vi "Photon Counter 11_21_2018.vi"(8 "error in (no error)":errorcluster) -> (0 "error out":errorcluster)   [LabVIEW 2015]
uses:
  Public/Typedefs/Gate Mode.ctl
  Public/Typedefs/Discriminator Output.ctl
  <vilib>/Instr/_visa.llb/VISA GPIB Control REN Mode.ctl
  <vilib>/DAQmx/read.llb/DAQmx Read (Analog 2D DBL NChan NSamp).vi
  <vilib>/DAQmx/read.llb/DAQmx Read (Analog 1D DBL NChan 1Samp).vi
  <vilib>/DAQmx/write.llb/DAQmx Write (Analog DBL 1Chan 1Samp).vi
  <vilib>/DAQmx/create/channels.llb/DAQmx Create Channel (AI-Voltage-Basic).vi
  <vilib>/DAQmx/create/channels.llb/DAQmx Create Channel (AO-Voltage-Basic).vi
  <vilib>/Waveform/WDTFileIO.llb/Export Waveforms To Spreadsheet File (1D).vi
  <vilib>/DAQmx/miscellaneous.llb/DAQmx Fill In Error Info.vi
  SR400.lvlib
panel:
  out "Trigger":bool
  out "PMT":dbl(graph)=0.36701612740637457
  out "Wavemeter":dbl(graph)=5.385889833071226
  in  "file path":path=path "C:/Users/physics/Desktop/tessttt.xls"
  out "Scanning":bool=TRUE
  out "Scan Finished":bool
  out "Current Period":dbl=26.0
  out "Counter A":dbl(graph)
  out "Counter B":dbl(graph)
  in  "Monitor":bool
  in  "Start Scan":bool caption="Start Monitored Scan"
  in  "Stop Scan":bool
  out "Scan Start Time":timestamp=timestamp(3418301700.0437126 s since 1904-01-01)
  out "Counter A":dbl(graph)=5052.0
  out "Counter B":dbl(graph)=5104.0
  in  "Read Buffer Data":bool
  in  "Query Status Byte":bool
  out "Scan Start Time":timestamp=timestamp(3611333596.390047 s since 1904-01-01)
  in  "GPIB Address":i32=23 min=0 max=30 step=1
  in  "Stop Unmonitored Scan":bool
  in  "Disc A Mode":T1
  in  "Disc B Mode":T1
  in  "Disc B Slope":enum16{"Rise", "Fall"}(ring)
  in  "Disc A Slope":enum16{"Rise", "Fall"}(ring)
  in  "Trigger Slope":enum16{"Rise", "Fall"}(ring)
  in  "Set Gate Widths":bool
  in  "Set Gate Mode":bool
  out "Current":dbl[unit]=0.5 caption="Current Dwell Time"
  in  "Setpoint":dbl[unit]=0.5 caption="Dwell Time Target" min=0.0 max=60.0 step=0.5 format="%#_1g"
  in  "Set Dwell Time":bool
  in  "Setpoint":i32=2000 caption="Number of Periods Target" min=0 max=2000 step=1
  out "Current":dbl=2000.0 caption="Number of Periods Current"
  in  "Set # Periods":bool
  in  "Scan End Mode":enum16{"Stop", "Start"}(ring)
  in  "Disc B Lvl":dbl=-0.012 format="%#_13g"
  in  "Disc A Lvl":dbl=-0.012 format="%#_13g"
  in  "Display Mode":enum16{"Continuous", "Hold"}(ring)
  in  "Initialize":bool
  in  "Internal / External":bool
  in  "Set Count Time":bool
  in  "Counter B Input":enum16{"10 MHz", "INPUT 1", "INPUT 2", "TRIG"}(ring)=enum."INPUT 1"
  in  "Counter A Input":enum16{"10 MHz", "INPUT 1", "INPUT 2", "TRIG"}(ring)=enum."INPUT 1"
  in  "Count Mode":T2(ring)
  in  "Trigger Level":dbl=1.25 format="%#_13g"
  in  "VISA Resource Name":refnum<visa-resource-name>="GPIB0::23::INSTR"
  in  "Photon Counter SR 400":T3={"Mode"=0, "Count Time"=0.5, "Trigger Frequency"=10000000.0, "Trigger External?"=FALSE, "Gate A Mode"=1, "Gate A Width"=0.0002, "Gate A Delay"=0.0001, "Gate B Mode"=1, "Gate B Width"=0.0001, "Gate B Delay"=0.0003} {"Mode" items=["A,B For T Preset", "A-B For T Preset", "A+B For T Preset", "A For B Preset"]; "Gate A Mode" items=["CW", "Fixed"]; "Gate B Mode" items=["CW", "Fixed"]}
  out "Update visible/hidden":bool
  out "Current":T4=enum."Fixed"
  out "Current":T4=enum."Fixed"
  in  "stop":bool
  in  "Read to\nControl":bool
  in  "Read":bool
  out "Actual":dbl=200000.00000000003
  out "Actual":dbl=100000.00000000001
  in  "Target":dbl=100000.00000000001 caption="Gate A Width Percent Target"
  in  "Target":dbl=200000.00000000003 caption="Gate A Percent Target"
  in  "Gate Width: Time / Percent":bool caption="Time/Percent"
  in  "Start / Middle":bool
  in  "Setpoint":T4=enum."Fixed" caption="Gate B Mode Target"
  in  "Setpoint":T4=enum."Fixed" caption="Gate A Mode Target"
  out "Current":dbl[unit]=10000000.0 caption="Trigger Freq"
  in  "Setpoint":dbl[unit]=10000000.0 caption="Trigger Freq. Target"
  in  "Set Time & Freq.":bool
  in  "# Triggers vs Freq/Time":bool
  out "Current":dbl=5000000.0 caption="External Trigger # Cycles Current" format="%^#_6g"
  in  "Setpoint":dbl=5000000.0 format="%^#_6g"
  in  "Set # of Triggers":bool
  in  "Setpoint":dbl[unit]=0.0001 caption="Gate B Width Target"
  in  "Setpoint":dbl[unit]=0.0002 caption="Gate A Width Target"
  out "Current":dbl[unit]=0.0002 format="%^#_6g"
  out "Current":dbl[unit]=0.0001 format="%^#_6g"
  out "Current":dbl[unit]=0.0003
  out "Current":dbl[unit]=0.0001
  in  "Setpoint":dbl[unit]=0.0003
  in  "Setpoint":dbl[unit]=0.0001 caption="Gate A Delay Target"
  in  "Set Gate Delays":bool
  in  "Start Unmonitored Scan":bool
  in  "Setpoint":dbl[unit]=0.5 caption="Count Time Target" min=0.0 step=0.5 format="%#_1f"
  out "Current":dbl[unit]=0.5 caption="Count Time Current" min=0.0 max=10000.0 step=1.0 format="%#_7g"
  # "SR400 Control Panel"
  # "Setup"
  # "Gates"
  # "Acquisition"
  # "Gate B Mode"
  # "# of Periods"
  # "Count Time"
  # "Gate A Mode"
  # "Gate A Width"
  # "Gate B Width"
  # "Dwell Time"
  # "Gate A Delay"
  # "Gate B Delay"
  # "Only Save\nAfter Scan"
  # "Discriminator/Trigger"
  # "Set values and initialize.\n\nSettings you can \"live\" update w/o initialization:\n        All Gate Params\n        Count Time (Only largest sig digit used)\n        Dwell Time (Only largest sig digit used)\n        External Trigger\n        # Periods\n\nSettings without a \"Set _____\" button need to be changed by initialization.\n\nAll variables are initialized, but \"live\" params do not show current value until you press the set button for that parameter.\n\n\"Read\" sets the \"Current\" indicators to what the hardware has set.\n\n\"Read to Control\" sets the \"Setpoint\" controls to the values from \"Read\""
  # "Warning, saving data clears chart histories"
  # "External Trigger # of Cycles/Freq"
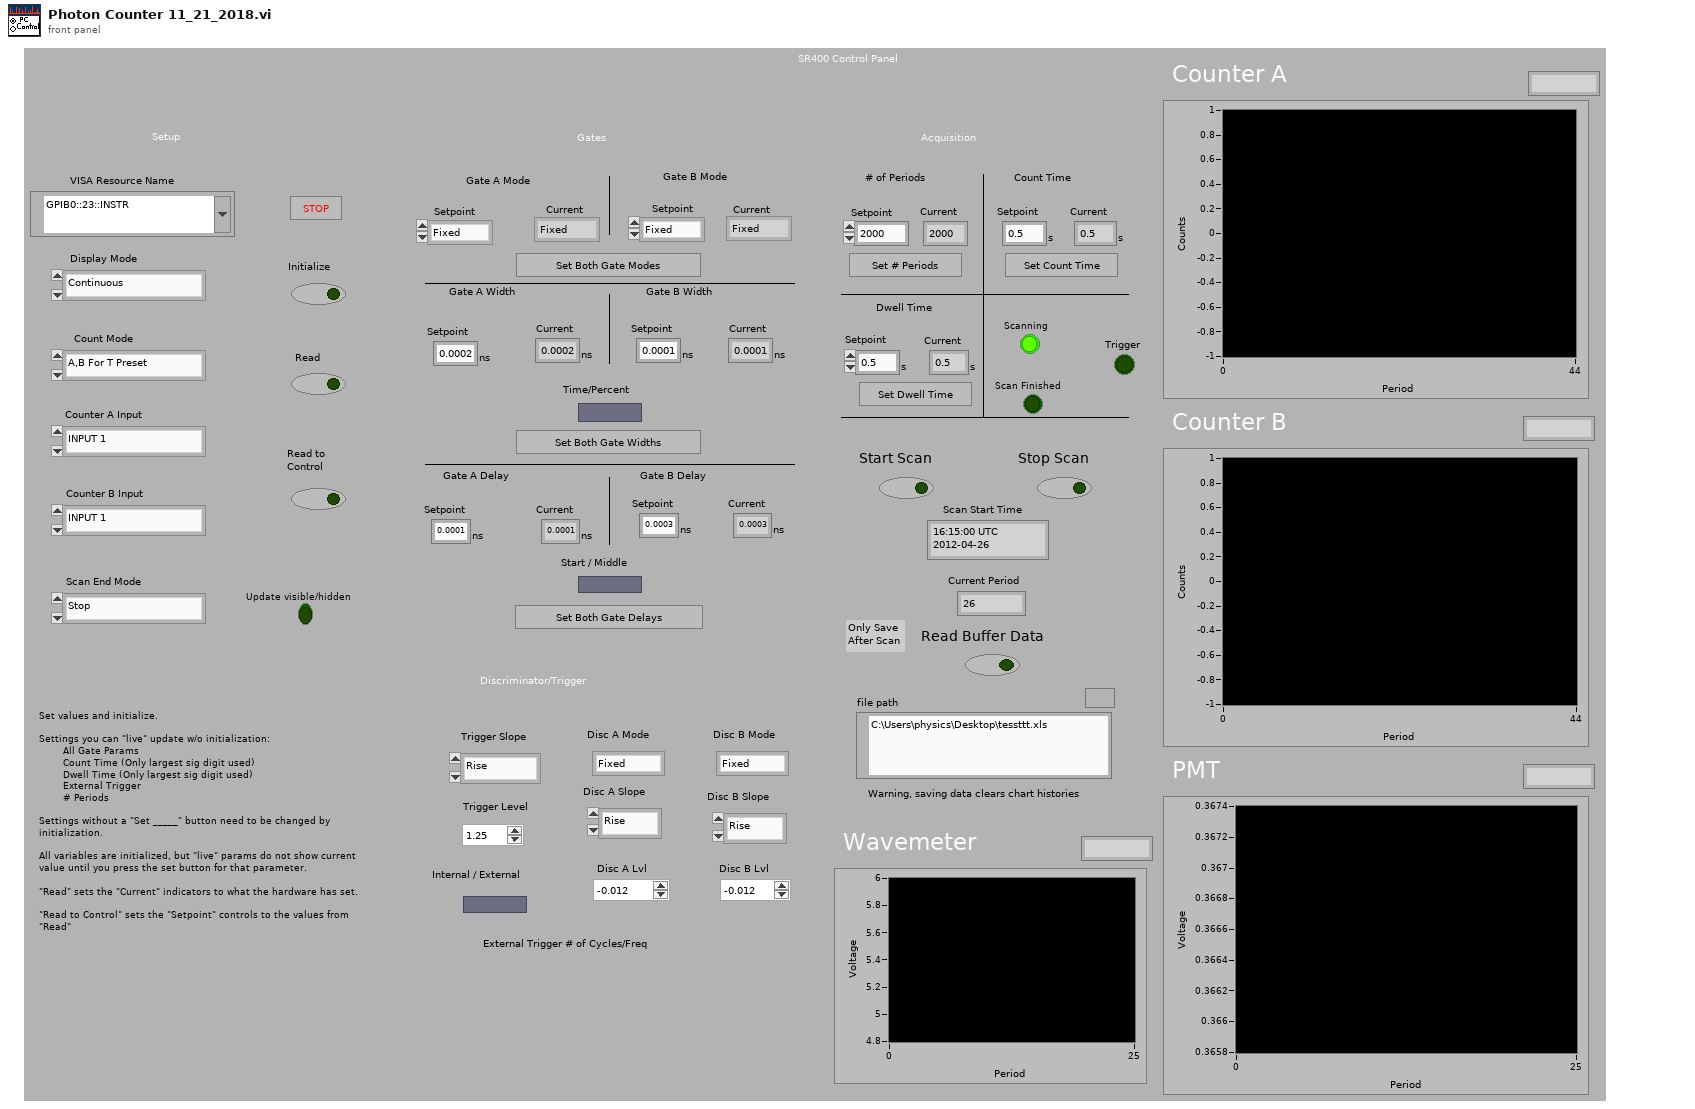
[diagram p1: front panel]
types:
  T1 = typedef "SR400.lvlib/Discriminator Output.ctl" = enum16{"Fixed", "Scan"}
  T2 = enum16{"A,B For T Preset", "A-B For T Preset", "A+B For T Preset", "A For B Preset"}
  T3 = cluster{"Mode":u16, "Count Time":dbl[unit], "Trigger Frequency":dbl[unit], "Trigger External?":bool, "Gate A Mode":u16, "Gate A Width":dbl[unit], "Gate A Delay":dbl[unit], "Gate B Mode":u16, "Gate B Width":dbl[unit], "Gate B Delay":dbl[unit]}
  T4 = typedef "SR400.lvlib/Gate Mode.ctl" = enum16{"CW", "Fixed", "Scan"}
  T5 = typedef "VISA GPIB Control REN Mode.ctl" = u16
  T6 = cluster{"Parameter Changed from front panel":bool, "Data Ready":bool, "Scan Finished":bool, "Counter Overrun":bool, "Rate Error":bool, "Recall Error":bool, "Service Request":bool, "Command Error":bool, "Triggered":bool, "Inhibited":bool, "Counting":bool}
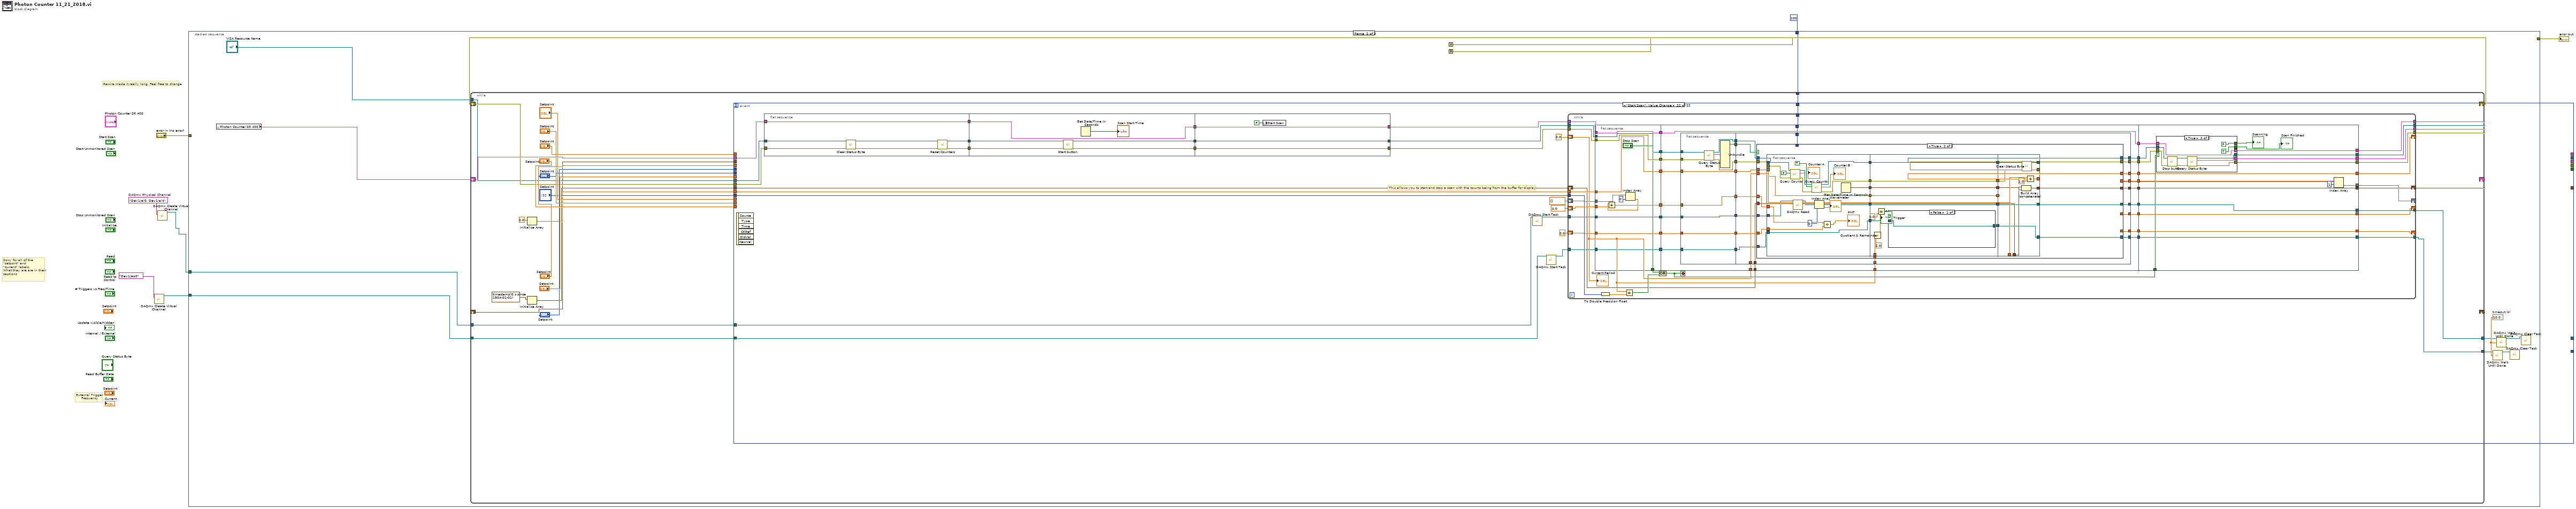
[diagram p0: block diagram]
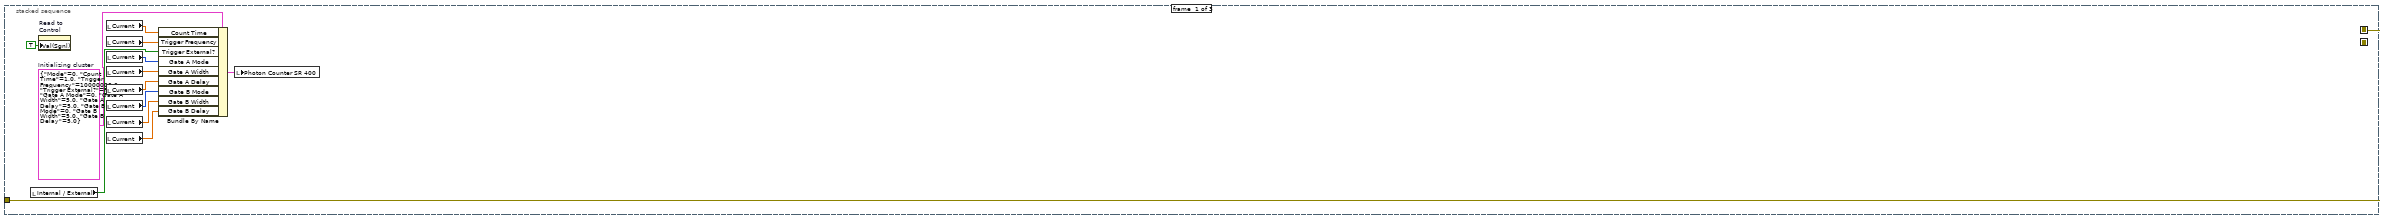
[diagram p2: hidden frame]
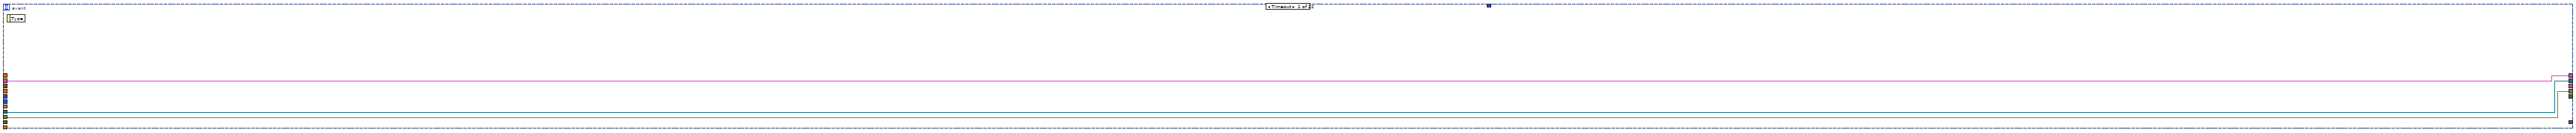
[diagram p3: hidden frame]
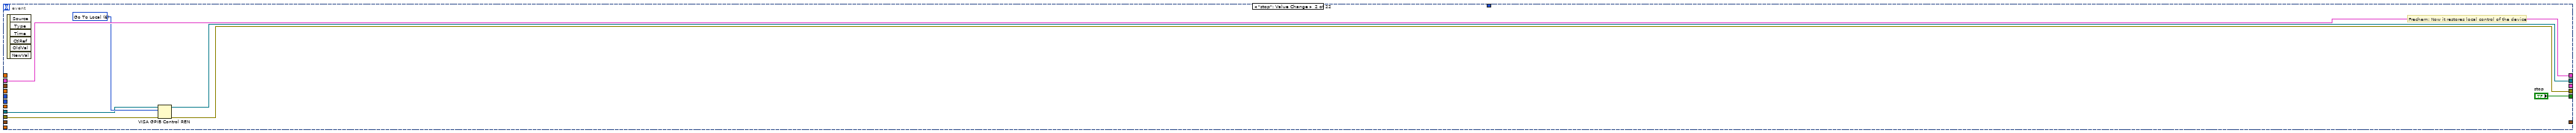
[diagram p4: hidden frame]
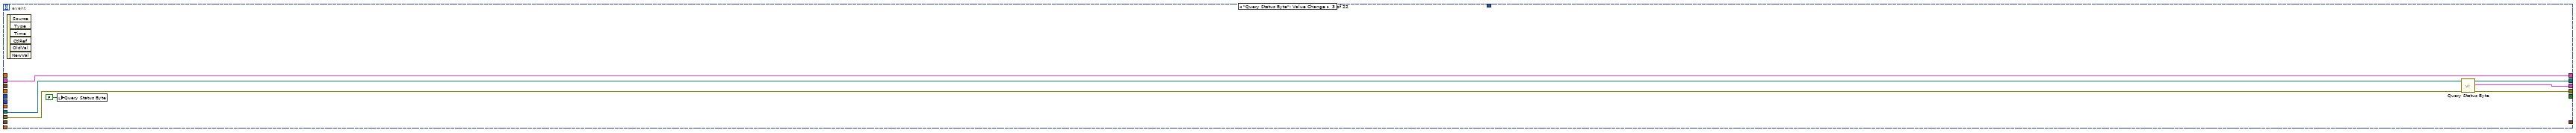
[diagram p5: hidden frame]
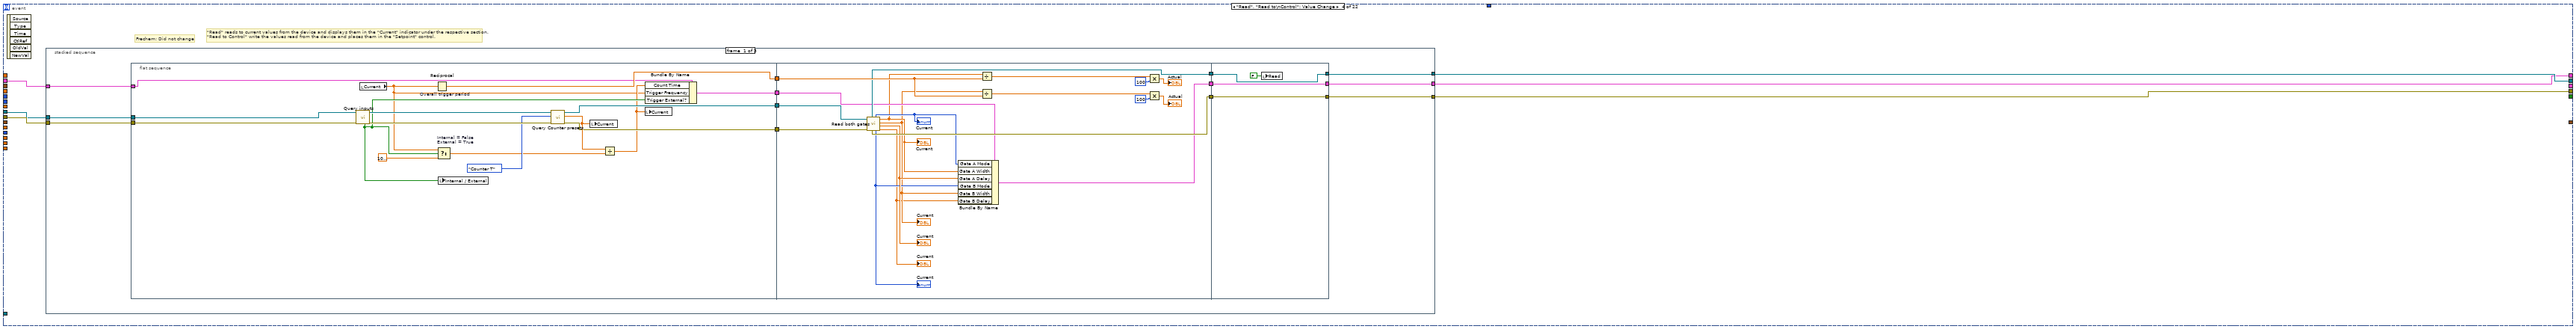
[diagram p6: hidden frame]
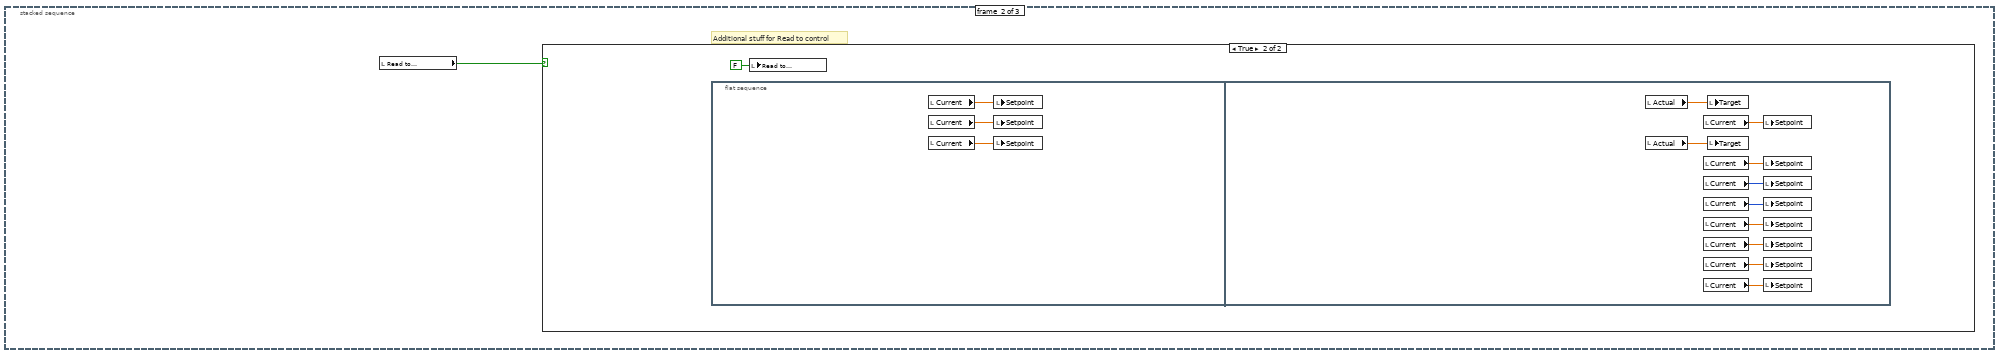
[diagram p7: hidden frame]
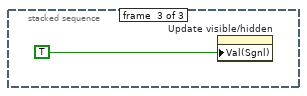
[diagram p9: hidden frame]
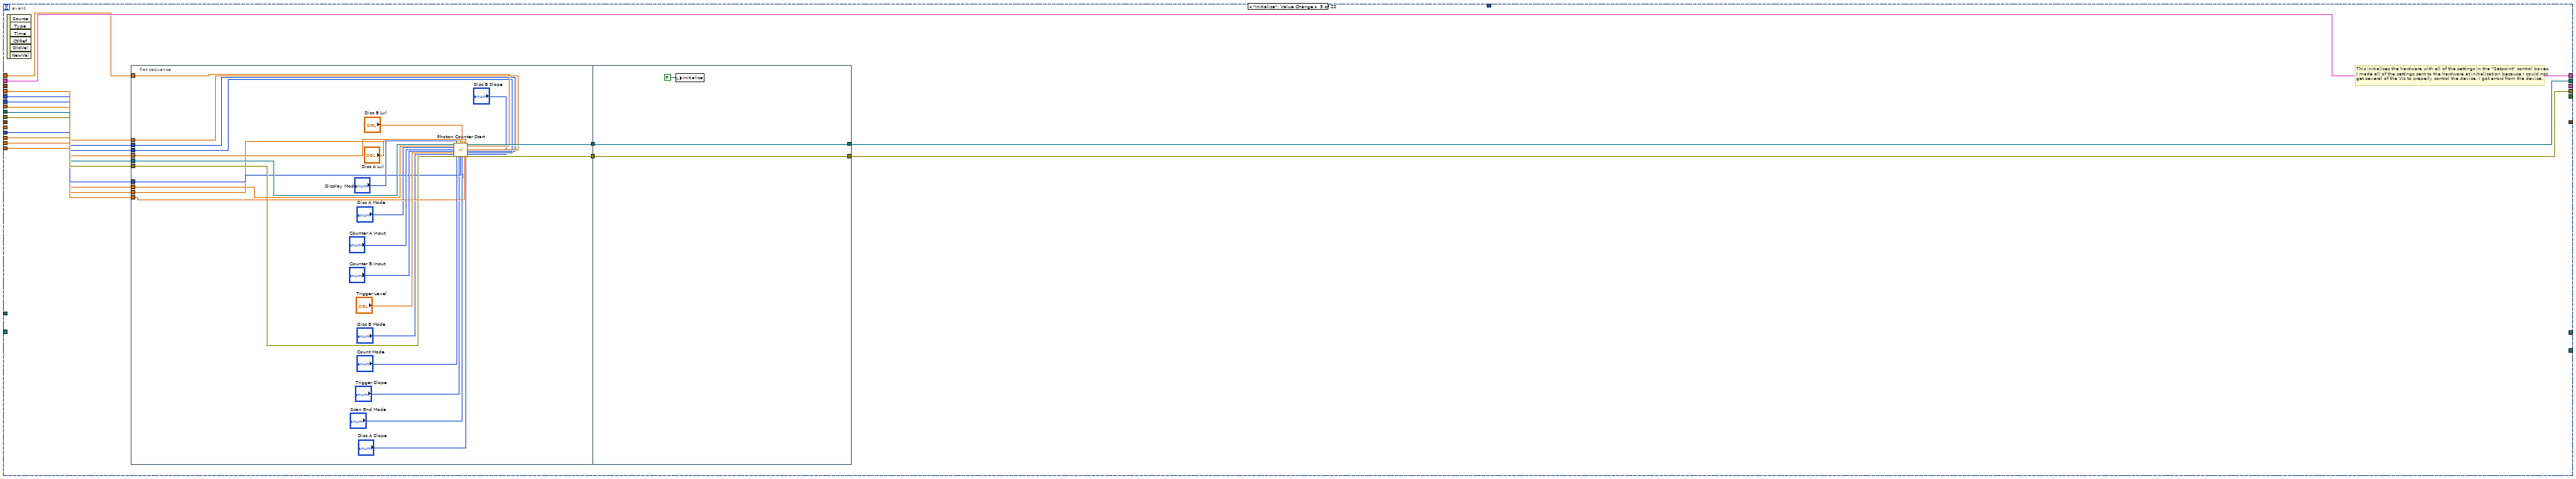
[diagram p10: hidden frame]
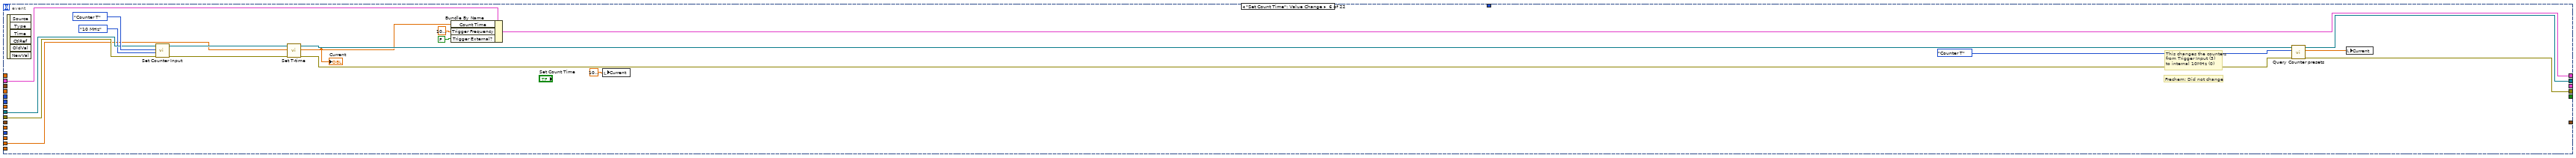
[diagram p11: hidden frame]
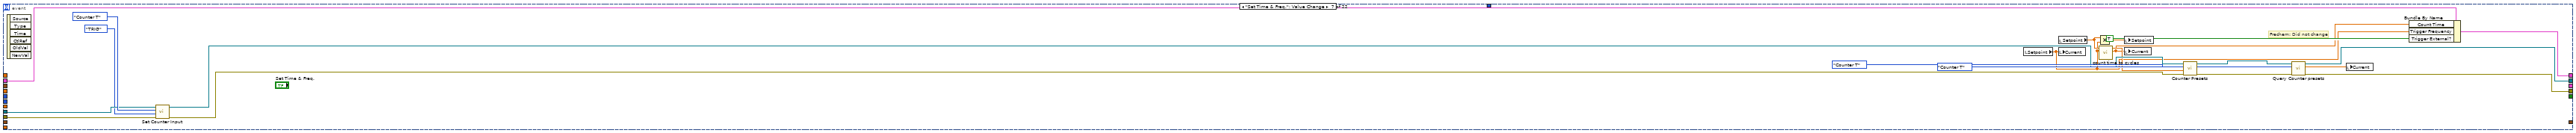
[diagram p12: hidden frame]
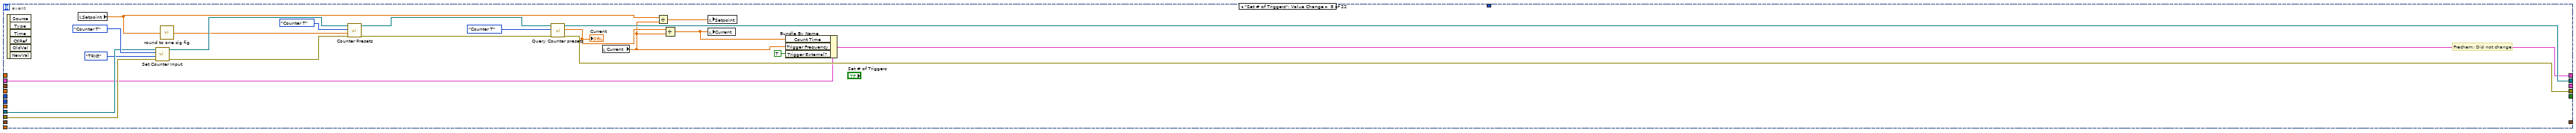
[diagram p13: hidden frame]
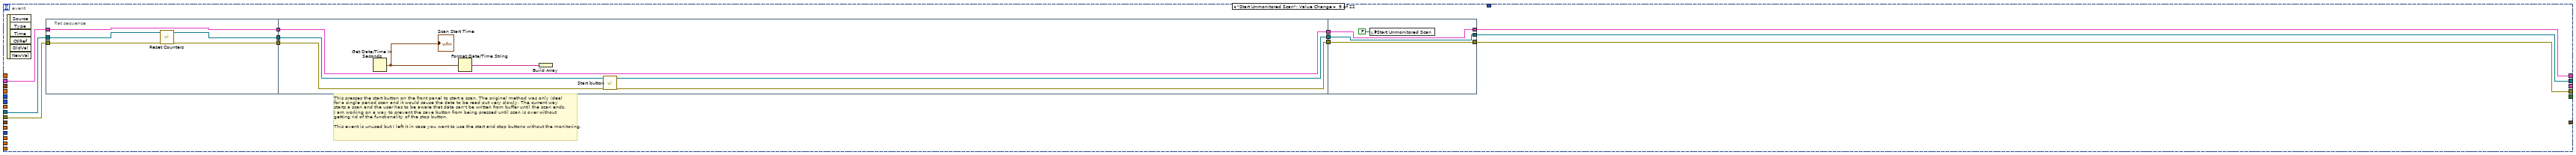
[diagram p14: hidden frame]
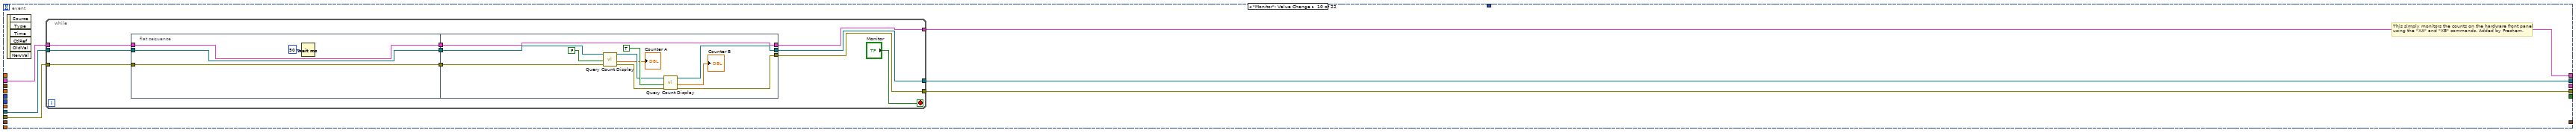
[diagram p15: hidden frame]
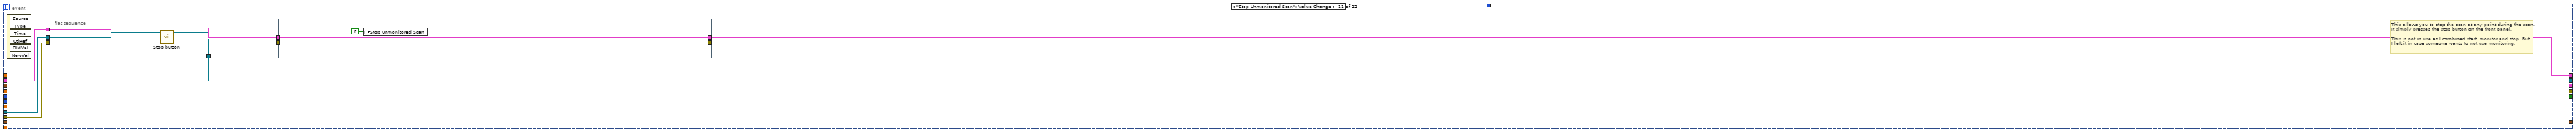
[diagram p16: hidden frame]
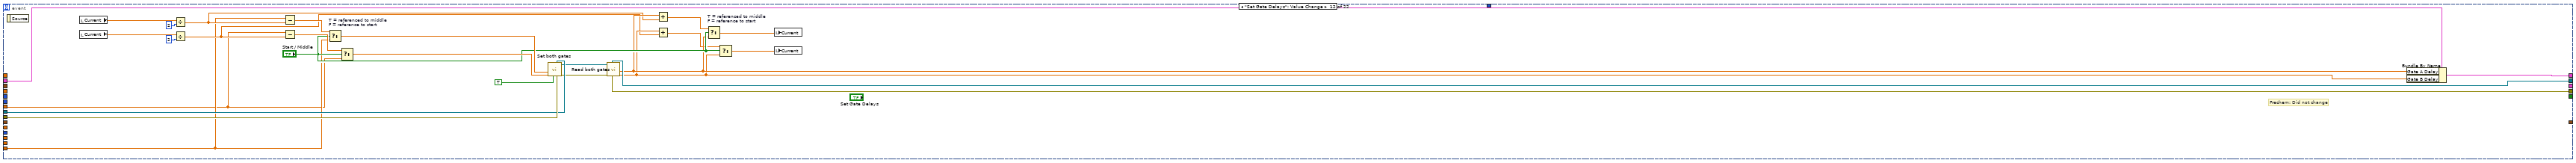
[diagram p17: hidden frame]
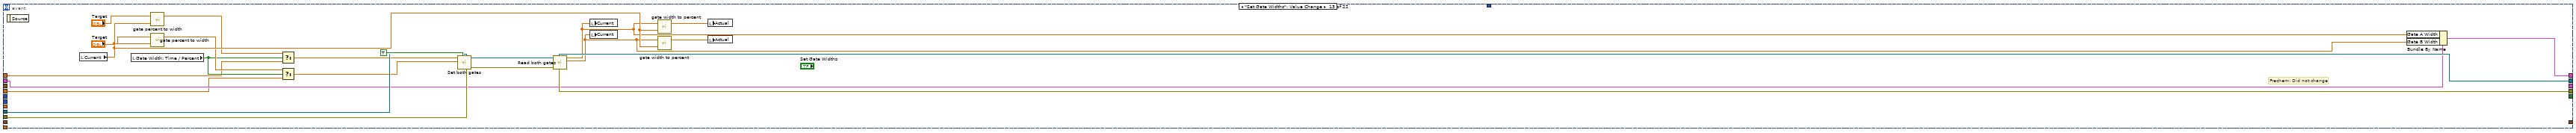
[diagram p18: hidden frame]
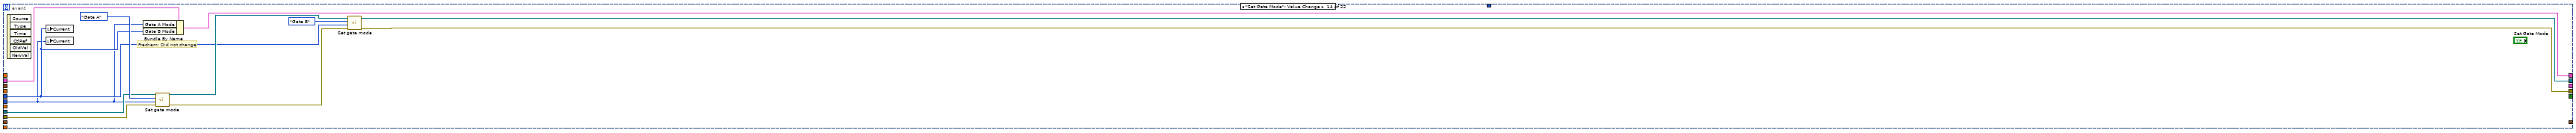
[diagram p19: hidden frame]
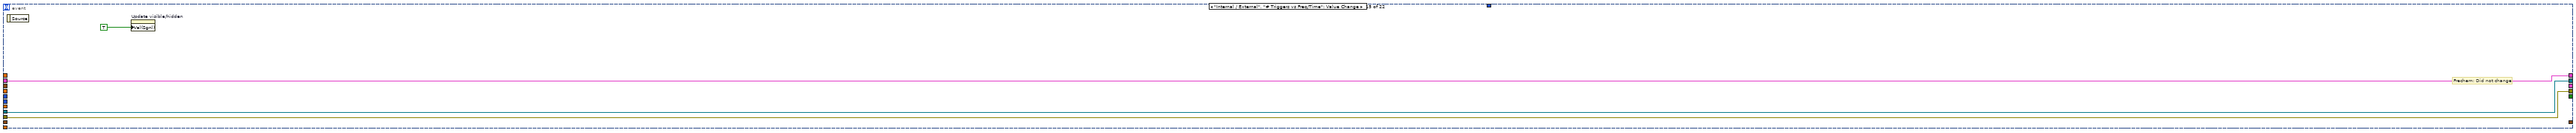
[diagram p20: hidden frame]
diagram:
  w4 = tag "Dev1/ai0, Dev1/ai4"  # DAQmx Physical Channel
  # "Rewire made it really long. Feel free to change"
  # "Sorry for all of the\n\"setpont\" and \n\"current\" labels. \nWhat they are are in their\ncaptions"
  # "External Trigger \n     Frequency"
  n1 = call-poly <vilib>:"DAQmx Create Virtual Channel.vi"("physical channels"=tag "Dev1/ao0") -> ("task out"=w1:refnum<k21>)  [unwired: 13 in, 1 out]
  n2 = call-poly <vilib>:"DAQmx Create Virtual Channel.vi"("physical channels"=w4) -> ("task out"=w3:refnum<k21>)  [unwired: 13 in, 1 out]
  n3 = stacked-sequence {
    seq-local: [w10 _ _] -> [_ w32 _]
    seq-local: [_ w31 _] -> [_ _ w874]
    tunnel: "error in (no error)" -> [w10 _ _]
    tunnel: [_ _ w874] -> w6
    tunnel: 100 ("number of samples per channel") -> [_ w28 _]
    tunnel: w3 -> [_ w27 _]
    tunnel: w1 -> [_ w26 _]
    frame #0 {
      w8 = T3 {"Mode"=0, "Count Time"=1.0, "Trigger Frequency"=10000000.0, "Trigger External?"=FALSE, "Gate A Mode"=0, "Gate A Width"=5.0, "Gate A Delay"=5.0, "Gate B Mode"=0, "Gate B Width"=5.0, "Gate B Delay"=5.0}  # Initializing cluster
      n4 = local read "Internal / External"() -> (w17:bool)
      n5 = property on="Read to\nControl" class="Bool (strict)"("Val(Sgnl)"=TRUE ("Value (Signaling)")) -> ()  [unwired: 2 in, 2 out]
      n6 = local read "Current"() -> (w19:dbl[unit])
      n7 = local read "Current"() -> (w18:dbl[unit])
      n8 = local read "Current"() -> (w16:T4)
      n9 = local read "Current"() -> (w15:dbl[unit])
      n10 = local read "Current"() -> (w14:dbl[unit])
      n11 = local read "Current"() -> (w11:T4)
      n12 = local read "Current"() -> (w12:dbl[unit])
      n13 = local read "Current"() -> (w13:dbl[unit])
      n14 = Bundle By Name(cluster=w8, "Count Time"=w19, "Trigger Frequency"=w18, "Trigger External?"=w17, "Gate A Mode"=w16, "Gate A Width"=w15, "Gate A Delay"=w14, "Gate B Mode"=w11, "Gate B Width"=w12, "Gate B Delay"=w13) -> (w9:T3)
      n15 = local write "Photon Counter SR 400"(w9) -> ()
    }
    frame #1 {
      w24 = 10.0  # timeout (s)
      n16 = local read "Photon Counter SR 400"() -> (w30:T3)
      n17 = while {
        shift-right: [w56] -> _
        shift-left: w30 -> [w55]
        shift-right: [w58] -> w31
        shift-left: w32 -> [w46]
        tunnel: "VISA Resource Name" -> [w45]
        shift-right: [w39] -> _
        shift-left: _ -> [w38]
        tunnel: w27 -> [w37]
        tunnel: w28 -> [w36]
        tunnel: w26 -> [w35]
        tunnel: [w34] -> w23
        tunnel: [w33] -> w21
        stop <- w57 stop-if-true
        n18 = Initialize Array(0.0 ("element")) -> (w42:dbl[])  [unwired: 1 in]
        n19 = Initialize Array(timestamp(0 s since 1904-01-01)) -> (w40:timestamp[])  [unwired: 1 in]
        n20 = event shown="[21] \"Start Scan\": Value Change" {
          selector: _ -> [_ _ _ _ _ _ _ _ _ _ _ _ _ _ _ _ _ _ _ _ _ _]
          dyn-events: _ -> [_ _ _ _ _ _ _ _ _ _ _ _ _ _ _ _ _ _ _ _ _ _]
          timeout: _ -> [_ _ _ _ _ _ _ _ _ _ _ _ _ _ _ _ _ _ _ _ _ _]
          tunnel: [w61 w63 w71 w80 w162 w212 w230 w254 w264 w289 w317 w344 w376 w386 w397 w400 w426 w459 w475 w482 w507 w586] -> _
          tunnel: w46 -> [w60 w66 w73 w82 w166 w203 w224 w246 w268 w288 w320 w358 w377 w390 w396 w398 w425 w458 w472 w488 w510 w589]
          tunnel: [w60 w65 w72 w79 w165 w211 w231 w253 w266 w290 _ w342 w375 w387 w396 w399 w425 w458 w474 w481 w509 w588] -> w59
          tunnel: w45 -> [w61 w64 w74 w81 w160 w204 w225 w247 w260 w287 w319 w357 w378 w391 w397 w400 w426 w459 w473 w489 w508 w590]
          tunnel: w55 -> [w62 w68 w76 w78 w161 w201 w219 w240 w262 w286 w318 w356 w364 w385 w395 w401 w427 w457 w471 w480 w506 w591]
          tunnel: [w62 w68 w76 w77 w161 w200 w218 w239 w261 w285 w316 w355 w363 w384 w395 w401 w427 w457 w471 w480 w505 w587] -> w56
          tunnel: [_ "stop" _ _ _ _ _ _ _ _ _ _ _ _ _ _ _ _ _ _ _ _] -> w57
          tunnel: "Setpoint" -> [_ _ _ _ w159 _ _ _ _ _ _ _ _ _ _ _ _ _ w470 _ w504 w582]
          tunnel: "Setpoint" -> [_ _ _ _ w158 _ _ _ _ _ _ _ w360 _ _ _ _ _ _ _ _ _]
          tunnel: "Setpoint" -> [_ _ _ _ w157 _ _ _ _ _ _ _ w359 _ _ _ _ _ _ _ _ _]
          tunnel: "Setpoint" -> [_ _ _ _ w156 _ _ _ _ _ _ w332 _ _ _ _ _ _ _ _ _ _]
          tunnel: "Setpoint" -> [_ _ _ _ w155 _ _ _ _ _ _ w331 _ _ _ _ _ _ _ _ _ _]
          tunnel: "Setpoint" -> [_ _ _ _ w154 w196 _ _ _ _ _ _ _ _ _ _ _ _ _ _ w492 _]
          tunnel: "Setpoint" -> [_ _ _ _ w152 _ _ _ _ _ _ _ _ w383 _ _ _ _ _ _ _ _]
          tunnel: "Setpoint" -> [_ _ _ _ w153 _ _ _ _ _ _ _ _ w382 _ _ _ _ _ _ _ _]
          tunnel: "Setpoint" -> [_ _ _ _ w151 _ _ _ _ _ _ _ _ _ _ _ _ _ _ w486 w493 _]
          tunnel: [_ _ w70 _ _ _ _ _ _ _ _ _ _ _ _ _ _ _ _ _ _ w585] -> _
          tunnel: w42 -> [_ _ _ _ _ _ _ _ _ _ _ _ _ _ _ _ _ _ _ _ _ w583]
          tunnel: w40 -> [_ _ _ _ _ _ _ _ _ _ _ _ _ _ _ _ _ _ _ _ _ w581]
          tunnel: [_ _ _ _ _ _ _ _ _ _ _ _ _ _ _ _ _ _ _ _ _ w580] -> w39
          tunnel: w38 -> [_ _ _ _ _ _ _ _ _ _ _ _ _ _ _ _ _ _ _ _ w494 _]
          tunnel: w37 -> [_ _ _ _ _ _ _ _ _ _ _ _ _ _ _ _ _ _ _ _ _ w575]
          tunnel: w36 -> [_ _ _ _ _ _ _ _ _ _ _ _ _ _ _ _ _ _ _ _ _ w579]
          tunnel: w35 -> [_ _ _ _ _ _ _ _ _ _ _ _ _ _ _ _ _ _ _ _ _ w573]
          tunnel: [_ _ _ _ _ _ _ _ _ _ _ _ _ _ _ _ _ _ _ _ _ w571] -> w34
          tunnel: [_ _ _ _ _ _ _ _ _ _ _ _ _ _ _ _ _ _ _ _ _ w570] -> w33
          event Timeout {
            n21 = event-data() -> ()  [unwired: 2 out]
          }
          event "stop": Value Change {
            w67 = T5 6 items=["Deassert REN", "Assert REN", "Go To Local; Deassert REN ", "Assert REN; Address Device", "Local Lockout (Addressed Devices)", "Local Lockout (This Device)", "Go To Local"] ("Mode")
            # "Frechem: Now it restores local control of the device"
            n22 = event-data() -> ()  [unwired: 7 out]
            n23 = VISA GPIB Control REN(8:w66, 10:w67, 11:w64) -> (0:w65:errorcluster, 3:w63:refnum<visa-resource-name>)
          }
          event "Query Status Byte": Value Change {
            n24 = event-data() -> ()  [unwired: 7 out]
            n25 = local write "Query Status Byte"(FALSE ("Read Channels")) -> ()
            n26 = call "Query Status Byte.vi"("error in (no error)"=w73, "VISA resource name"=w74) -> ("error out"=w72:errorcluster, "Status Register"=w70:T6, "VISA resource name out"=w71:refnum<visa-resource-name>)  [unwired: 7 in]
          }
          event "Read", "Read to\nControl": Value Change {
            # "Frechem: Did not change"
            # "\"Read\" reads to current values from the device and displays them in the \"Current\" indicator under the respective section.\n\"Read to Control\" write the values read from the device and places them in the \"Setpoint\" control."
            n27 = event-data() -> ()  [unwired: 7 out]
            n28 = stacked-sequence {
              tunnel: w82 -> [w94 _ _]
              tunnel: w81 -> [w95 _ _]
              tunnel: [w90 _ _] -> w80
              tunnel: [w88 _ _] -> w79
              tunnel: w78 -> [w86 _ _]
              tunnel: [w84 _ _] -> w77
              frame #0 {
                n29 = flat-sequence {
                  tunnel: w95 -> [w111]
                  tunnel: w94 -> [w108]
                  tunnel: [w104] -> w93
                  tunnel: [w103] -> w92
                  tunnel: [w102] -> w91
                  tunnel: w86 -> [w100]
                  tunnel: [w96] -> w85
                  tunnel: w93 -> [w124]
                  tunnel: w92 -> [w123]
                  tunnel: w91 -> [w122]
                  tunnel: [w121] -> w89
                  tunnel: [w120] -> w87
                  tunnel: w85 -> [w119]
                  tunnel: [w112] -> w83
                  tunnel: [w133] -> w90
                  tunnel: w89 -> [w133]
                  tunnel: [w132] -> w88
                  tunnel: w87 -> [w132]
                  tunnel: [w131] -> w84
                  tunnel: w83 -> [w131]
                  frame #0 {
                    n30 = call "Query inputs.vi"("error in (no error)"=w108, "VISA resource name"=w111) -> ("error out"=w109:errorcluster, "VISA resource name out"=w110:refnum<visa-resource-name>, "Externally-triggered?"=w99:bool)  [unwired: 7 out]
                    n31 = local read "Current"() -> (w97:dbl[unit])
                    n32 = Reciprocal "Overall trigger period"(x=w97) -> (1/x=w102:dbl[unit])
                    n33 = Select "Internal = False\nExternal = True"(t=w97, s=w99, f=dbl[unit] 10000000.0 ("freq")) -> (s? t:f=w106:dbl[unit])
                    n34 = local write "Internal / External"(w99) -> ()
                    n35 = call "Query Counter presets.vi"("error in (no error)"=w109, "Counter (Def: T)"=enum16{"Invalid", "Counter B", "Counter T"}."Counter T" ("i (0)"), "VISA resource name"=w110) -> ("error out"=w103:errorcluster, "Number of triggers"=w105:dbl, "VISA resource name out"=w104:refnum<visa-resource-name>)  [unwired: 6 out]
                    n36 = local write "Current"(w105) -> ()
                    n37 = Divide(x=w105, y=w106) -> (x/y=w98:dbl[unit])
                    n38 = Bundle By Name(cluster=w100, "Count Time"=w98, "Trigger Frequency"=w97, "Trigger External?"=w99) -> (w96:T3)
                    n39 = local write "Current"(w98) -> ()
                  }
                  frame #1 {
                    n40 = call "Read both gates.vi"("error in (no error)"=w123, "VISA resource name"=w124) -> ("Gate B Delay"=w113:dbl[unit], "Gate A Delay"=w116:dbl[unit], "Gate B Width"=w114:dbl[unit], "Gate A Width"=w117:dbl[unit], "Current mode B"=w115:enum16{"CW", "Fixed", "Scan"}, "Current mode A"=w118:enum16{"CW", "Fixed", "Scan"}, "error out"=w120:errorcluster, "VISA resource name out"=w121:refnum<visa-resource-name>)  [unwired: 2 out]
                    "Current" <- w114
                    "Current" <- w117
                    "Current" <- w116
                    "Current" <- w113
                    "Current" <- w118
                    "Current" <- w115
                    n41 = Bundle By Name(cluster=w119, "Gate A Mode"=w118, "Gate A Width"=w117, "Gate A Delay"=w116, "Gate B Mode"=w115, "Gate B Width"=w114, "Gate B Delay"=w113) -> (w112:T3)
                    n42 = Divide(x=w117, y=w122) -> (x/y=w126:dbl)
                    n43 = Divide(x=w114, y=w122) -> (x/y=w128:dbl)
                    n44 = Multiply(x=w126, y=i8 100) -> (x*y=→"Actual":dbl)
                    n45 = Multiply(x=w128, y=i8 100) -> (x*y=→"Actual":dbl)
                  }
                  frame #2 {
                    n46 = local write "Read"(FALSE ("Read")) -> ()
                  }
                }
              }
              frame #1 {
                # "Additional stuff for Read to control"
                n47 = local read "Read to\nControl"() -> (w135:bool)
                n48 = case shown="True" w135 {
                  frame False {
                  }
                  frame True {
                    n49 = flat-sequence {
                      frame #0 {
                        n50 = local read "Current"() -> (w138:dbl)
                        n51 = local read "Current"() -> (w137:dbl[unit])
                        n52 = local read "Current"() -> (w139:dbl[unit])
                        n53 = local write "Setpoint"(w138) -> ()
                        n54 = local write "Setpoint"(w137) -> ()
                        n55 = local write "Setpoint"(w139) -> ()
                      }
                      frame #1 {
                        n56 = local read "Actual"() -> (w146:dbl)
                        n57 = local read "Actual"() -> (w148:dbl)
                        n58 = local read "Current"() -> (w141:dbl[unit])
                        n59 = local read "Current"() -> (w142:dbl[unit])
                        n60 = local read "Current"() -> (w144:T4)
                        n61 = local read "Current"() -> (w143:T4)
                        n62 = local read "Current"() -> (w147:dbl[unit])
                        n63 = local read "Current"() -> (w145:dbl[unit])
                        n64 = local read "Current"() -> (w149:dbl[unit])
                        n65 = local read "Current"() -> (w140:dbl[unit])
                        n66 = local write "Target"(w146) -> ()
                        n67 = local write "Target"(w148) -> ()
                        n68 = local write "Setpoint"(w141) -> ()
                        n69 = local write "Setpoint"(w142) -> ()
                        n70 = local write "Setpoint"(w144) -> ()
                        n71 = local write "Setpoint"(w143) -> ()
                        n72 = local write "Setpoint"(w147) -> ()
                        n73 = local write "Setpoint"(w145) -> ()
                        n74 = local write "Setpoint"(w149) -> ()
                        n75 = local write "Setpoint"(w140) -> ()
                      }
                    }
                    n76 = local write "Read to\nControl"(FALSE ("Read to Control")) -> ()
                  }
                }
              }
              frame #2 {
                n77 = property on="Update visible/hidden" class="Bool (strict)"("Val(Sgnl)"=TRUE ("Value (Signaling)")) -> ()  [unwired: 2 in, 2 out]
              }
            }
          }
          event "Initialize": Value Change {
            # "This initializes the hardware with all of the settings in the \"Setpoint\" control boxes.\nI made all of the settings sent to the hardware at initialization because I could not \nget several of the VIs to preperly control the device. I got errors from the device."
            n78 = event-data() -> ()  [unwired: 7 out]
            n79 = flat-sequence {
              tunnel: w166 -> [w192]
              tunnel: [w191] -> w164
              tunnel: [w190] -> w163
              tunnel: w160 -> [w189]
              tunnel: w159 -> [w180]
              tunnel: w158 -> [w179]
              tunnel: w157 -> [w178]
              tunnel: w156 -> [w177]
              tunnel: w155 -> [w176]
              tunnel: w154 -> [w175]
              tunnel: w153 -> [w174]
              tunnel: w152 -> [w173]
              tunnel: w151 -> [w172]
              tunnel: [w194] -> w165
              tunnel: [w195] -> w162
              tunnel: w164 -> [w195]
              tunnel: w163 -> [w194]
              frame #0 {
                n80 = call "Photon Counter Start.vi"("VISA resource name"=w189, "Dwell Time"=w172, "Disc A Mode"="Disc A Mode", "Count A Input"="Counter A Input", "Count B Input"="Counter B Input", "Trigger Level"="Trigger Level", "Disc B Mode"="Disc B Mode", "errorIN"=w192, "Display Mode"="Display Mode", "Count Mode"="Count Mode", "Trigger Slope"="Trigger Slope", "Disc A Lvl"="Disc A Lvl", "# of periods"=w180, "Disc B Lvl"="Disc B Lvl", "Scan End Mode"="Scan End Mode", "Count Time Set"=w175, "Gate A Delay (def: 0 s)"=w177, "Gate B Delay (def: 0 s)"=w176, "Disc A\nSlope"="Disc A Slope", "Gate A Width (def: 0 s)"=w178, "Gate B Width (def: 0 s)"=w179, "Gate B Mode"=w173, "Gate A Mode"=w174, "Disc B\nSlope"="Disc B Slope") -> ("VISA resource name out"=w191:refnum<visa-resource-name>, "errorOUT"=w190:errorcluster)  [unwired: 2 in]
              }
              frame #1 {
                n81 = local write "Initialize"(FALSE ("Re-initialize")) -> ()
              }
            }
          }
          event "Set Count Time": Value Change {
            # "Frechem: Did not change"
            # "This changes the counters\nfrom Trigger Input (3)\nto internal 10MHz (0)"
            n82 = event-data() -> ()  [unwired: 7 out]
            n83 = call "Set Counter Input.vi"("error in (no error)"=w203, "Input (def: 10 MHz)"=enum16{"10 MHz", "INPUT 1", "INPUT 2", "TRIG"}."10 MHz" ("n (0.000000)"), "Counter (def: A)"=enum16{"Counter A", "Counter B", "Counter T"}."Counter T" ("i (0) 2"), "VISA resource name"=w204) -> ("error out"=w206:errorcluster, "VISA resource name out"=w205:refnum<visa-resource-name>)  [unwired: 6 out]
            n84 = call "Set T-time.vi"("errorIN"=w206, "Count Time Set"=w196, "VISA resource name"=w205) -> ("errorOUT"=w207:errorcluster, "ttimeOUT"=w199:dbl[unit], "VISA resource name out"=w210:refnum<visa-resource-name>)  [unwired: 4 out]
            "Current" <- w199
            n85 = Bundle By Name(cluster=w201, "Count Time"=w199, "Trigger Frequency"=dbl[unit] 10000000.0, "Trigger External?"=FALSE) -> (w200:T3)
            n86 = local write "Current"(dbl[unit] 10000000.0 ("freq")) -> ()
            n87 = call "Query Counter presets.vi"("error in (no error)"=w207, "Counter (Def: T)"=enum16{"Invalid", "Counter B", "Counter T"}."Counter T" ("i (0)"), "VISA resource name"=w210) -> ("error out"=w211:errorcluster, "Number of triggers"=w213:dbl, "VISA resource name out"=w212:refnum<visa-resource-name>)  [unwired: 6 out]
            n88 = local write "Current"(w213) -> ()
          }
          event "Set Time & Freq.": Value Change {
            # "Frechem: Did not change"
            n89 = event-data() -> ()  [unwired: 7 out]
            n90 = call "Set Counter Input.vi"("error in (no error)"=w224, "Input (def: 10 MHz)"=enum16{"10 MHz", "INPUT 1", "INPUT 2", "TRIG"}."TRIG" ("n (0.000000)"), "Counter (def: A)"=enum16{"Counter A", "Counter B", "Counter T"}."Counter T" ("i (0) 2"), "VISA resource name"=w225) -> ("error out"=w226:errorcluster, "VISA resource name out"=w227:refnum<visa-resource-name>)  [unwired: 6 out]
            n91 = local read "Setpoint"() -> (w215:dbl[unit])
            n92 = local read "Setpoint"() -> (w220:dbl[unit])
            n93 = local write "Current"(w215) -> ()
            n94 = Multiply(x=w220, y=w215) -> (x*y=w221:dbl)
            n95 = call "count time to cycles.vi"("Trigger Freq"=w215, "Count Time Set"=w220) -> ("Count Time Current"=w216:dbl[unit], "Number of triggers"=w222:dbl)  [unwired: 3 in, 1 out]
            n96 = local write "Setpoint"(w221) -> ()
            n97 = local write "Current"(w216) -> ()
            n98 = call "Counter Presets.vi"("error in (no error)"=w226, "Number of triggers"=w222, "Counter (Def: T)"=enum16{"Invalid", "Counter B", "Counter T"}."Counter T" ("i (0) 2"), "VISA resource name"=w227) -> ("error out"=w232:errorcluster, "VISA resource name out"=w229:refnum<visa-resource-name>)  [unwired: 6 out]
            n99 = call "Query Counter presets.vi"("error in (no error)"=w232, "Counter (Def: T)"=enum16{"Invalid", "Counter B", "Counter T"}."Counter T" ("i (0)"), "VISA resource name"=w229) -> ("error out"=w231:errorcluster, "Number of triggers"=w233:dbl, "VISA resource name out"=w230:refnum<visa-resource-name>)  [unwired: 6 out]
            n100 = local write "Current"(w233) -> ()
            n101 = Bundle By Name(cluster=w219, "Count Time"=w216, "Trigger Frequency"=w215, "Trigger External?"=TRUE) -> (w218:T3)
          }
          event "Set # of Triggers": Value Change {
            # "Frechem: Did not change"
            n102 = event-data() -> ()  [unwired: 7 out]
            n103 = local read "Setpoint"() -> (w244:dbl)
            n104 = call "Set Counter Input.vi"("error in (no error)"=w246, "Input (def: 10 MHz)"=enum16{"10 MHz", "INPUT 1", "INPUT 2", "TRIG"}."TRIG" ("n (0.000000)"), "Counter (def: A)"=enum16{"Counter A", "Counter B", "Counter T"}."Counter T" ("i (0) 2"), "VISA resource name"=w247) -> ("error out"=w248:errorcluster, "VISA resource name out"=w249:refnum<visa-resource-name>)  [unwired: 6 out]
            n105 = call "round to one sig fig.vi"("input number"=w244) -> ("rounded to 1 sig fig"=w242:dbl)
            n106 = call "Counter Presets.vi"("error in (no error)"=w248, "Number of triggers"=w242, "Counter (Def: T)"=enum16{"Invalid", "Counter B", "Counter T"}."Counter T" ("i (0) 2"), "VISA resource name"=w249) -> ("error out"=w252:errorcluster, "VISA resource name out"=w251:refnum<visa-resource-name>)  [unwired: 6 out]
            n107 = call "Query Counter presets.vi"("error in (no error)"=w252, "Counter (Def: T)"=enum16{"Invalid", "Counter B", "Counter T"}."Counter T" ("i (0)"), "VISA resource name"=w251) -> ("error out"=w253:errorcluster, "Number of triggers"=w241:dbl, "VISA resource name out"=w254:refnum<visa-resource-name>)  [unwired: 6 out]
            "Current" <- w241
            n108 = local read "Current"() -> (w236:dbl[unit])
            n109 = Divide(x=w244, y=w236) -> (x/y=w243:dbl[unit])
            n110 = Divide(x=w241, y=w236) -> (x/y=w238:dbl[unit])
            n111 = local write "Setpoint"(w243) -> ()
            n112 = local write "Current"(w238) -> ()
            n113 = Bundle By Name(cluster=w240, "Count Time"=w238, "Trigger Frequency"=w236, "Trigger External?"=TRUE) -> (w239:T3)
          }
          event "Start Unmonitored Scan": Value Change {
            # "This presses the start button on the front panel to start a scan. The original method was only ideal\nfor a single period scan and it would cause the data to be read out very slowly. The current way \nstarts a scan and the user has to be aware that data can't be written from buffer until the scan ends.\nI am working on a way to prevent the save button from being pressed until scan is over without \ngetting rid of the functionality of the stop button.\n\nThis event is unused but I left it in case you want to use the start and stop buttons without the monitoring."
            n114 = event-data() -> ()  [unwired: 7 out]
            n115 = flat-sequence {
              tunnel: w262 -> [w273]
              tunnel: w260 -> [w272]
              tunnel: w268 -> [w270]
              tunnel: [w269] -> w259
              tunnel: [w271] -> w258
              tunnel: [w273] -> w257
              tunnel: [w279] -> w267
              tunnel: [w277] -> w265
              tunnel: [w276] -> w263
              tunnel: w259 -> [w280]
              tunnel: w258 -> [w278]
              tunnel: w257 -> [w276]
              tunnel: [w281] -> w266
              tunnel: w267 -> [w281]
              tunnel: w265 -> [w282]
              tunnel: [w282] -> w264
              tunnel: [w283] -> w261
              tunnel: w263 -> [w283]
              frame #0 {
                n116 = call "Reset Counters.vi"("error in (no error)"=w270, "VISA resource name"=w272) -> ("error out"=w269:errorcluster, "VISA resource name out"=w271:refnum<visa-resource-name>)  [unwired: 8 in]
              }
              frame #1 {
                n117 = Get Date/Time In Seconds() -> (seconds since 1Jan1904=w275:timestamp)
                "Scan Start Time" <- w275
                n118 = Format Date/Time String(seconds (now)=w275) -> (date/time string=w274:string)  [unwired: 2 in]
                n119 = Build Array(w274) -> ()  [unwired: 1 out]
                n120 = call "Start button.vi"("error in (no error)"=w280, "VISA resource name"=w278) -> ("error out"=w279:errorcluster, "VISA resource name out"=w277:refnum<visa-resource-name>)  [unwired: 8 in]
              }
              frame #2 {
                n121 = local write "Start Unmonitored Scan"(FALSE ("Read Channels")) -> ()
              }
            }
          }
          event "Monitor": Value Change {
            # "This simply monitors the counts on the hardware front panel\nusing the \"XA\" and \"XB\" commands. Added by Frechem."
            n122 = event-data() -> ()  [unwired: 7 out]
            n123 = while {
              tunnel: w286 -> [w293]
              tunnel: [w292] -> w285
              tunnel: w287 -> [w294]
              tunnel: [w296] -> w289
              tunnel: w288 -> [w295]
              tunnel: [w297] -> w290
              stop <- "Monitor" stop-if-true
              n124 = flat-sequence {
                tunnel: w294 -> [w303]
                tunnel: [w303] -> w300
                tunnel: w295 -> [w302]
                tunnel: [w302] -> w299
                tunnel: w293 -> [w301]
                tunnel: [w301] -> w298
                tunnel: w300 -> [w307]
                tunnel: w299 -> [w306]
                tunnel: w298 -> [w305]
                tunnel: [w309] -> w296
                tunnel: [w308] -> w297
                tunnel: [w305] -> w292
                frame #0 {
                  n125 = Wait (ms)(milliseconds to wait=u32 50) -> ()  [unwired: 1 out]
                }
                frame #1 {
                  n126 = call "Query Count Display.vi"("error in (no error)"=w306, "Read B?"=FALSE, "VISA resource name"=w307) -> ("error out"=w314:errorcluster, "Counts"=→"Counter A":dbl, "VISA resource name out"=w312:refnum<visa-resource-name>)  [unwired: 6 in]
                  n127 = call "Query Count Display.vi"("error in (no error)"=w314, "Read B?"=TRUE, "VISA resource name"=w312) -> ("error out"=w308:errorcluster, "Counts"=→"Counter B":dbl, "VISA resource name out"=w309:refnum<visa-resource-name>)  [unwired: 6 in]
                }
              }
            }
          }
          event "Stop Unmonitored Scan": Value Change {
            # "This allows you to stop the scan at any point during the scan. \nIt simply presses the stop button on the front panel.\n\nThis is not in use as I combined start, monitor and stop. But, \nI left it in case someone wants to not use monitoring."
            n128 = event-data() -> ()  [unwired: 7 out]
            n129 = flat-sequence {
              tunnel: w320 -> [w326]
              tunnel: w318 -> [w325]
              tunnel: [w323] -> w322
              tunnel: [w325] -> w321
              tunnel: w319 -> [w327]
              tunnel: [w324] -> w317
              tunnel: [w329] -> w316
              tunnel: [w330] -> _
              tunnel: w322 -> [w330]
              tunnel: w321 -> [w329]
              frame #0 {
                n130 = call "Stop button.vi"("error in (no error)"=w326, "VISA resource name"=w327) -> ("error out"=w323:errorcluster, "VISA resource name out"=w324:refnum<visa-resource-name>)  [unwired: 8 in]
              }
              frame #1 {
                n131 = local write "Stop Unmonitored Scan"(FALSE ("Read Channels")) -> ()
              }
            }
          }
          event "Set Gate Delays": Value Change {
            # "Frechem: Did not change"
            n132 = event-data() -> ()  [unwired: 2 out]
            n133 = local read "Current"() -> (w353:dbl[unit])
            n134 = local read "Current"() -> (w352:dbl[unit])
            n135 = Divide(x=w353, y=2) -> (x/y=w333:dbl[unit])
            n136 = Divide(x=w352, y=2) -> (x/y=w334:dbl[unit])
            n137 = Subtract(x=w332, y=w333) -> (x-y=w349:dbl[unit])
            n138 = Subtract(x=w331, y=w334) -> (x-y=w347:dbl[unit])
            n139 = Select "T = referenced to middle\nF = reference to start"(t=w349, s="Start / Middle", f=w332) -> (s? t:f=w346:dbl[unit])
            n140 = Select(t=w347, s="Start / Middle", f=w331) -> (s? t:f=w348:dbl[unit])
            n141 = call "Set both gates.vi"("Error In"=w358, "VISA resource name"=w357, "Set Delay?"=TRUE, "gatedelayoffsetB"=w348, "gatedelayoffsetA"=w346) -> ("Error Out"=w343:errorcluster, "VISA resource name out"=w345:refnum<visa-resource-name>)  [unwired: 3 in, 2 out]
            n142 = call "Read both gates.vi"("error in (no error)"=w343, "VISA resource name"=w345) -> ("Gate B Delay"=w339:dbl[unit], "Gate A Delay"=w340:dbl[unit], "error out"=w342:errorcluster, "VISA resource name out"=w344:refnum<visa-resource-name>)  [unwired: 6 out]
            n143 = Add(x=w340, y=w333) -> (x+y=w338:dbl[unit])
            n144 = Add(x=w339, y=w334) -> (x+y=w337:dbl[unit])
            n145 = Select "T = referenced to middle\nF = reference to start"(t=w338, s="Start / Middle", f=w340) -> (s? t:f=w336:dbl[unit])
            n146 = Select(t=w337, s="Start / Middle", f=w339) -> (s? t:f=w335:dbl[unit])
            n147 = local write "Current"(w336) -> ()
            n148 = local write "Current"(w335) -> ()
            n149 = Bundle By Name(cluster=w356, "Gate A Delay"=w340, "Gate B Delay"=w339) -> (w355:T3)
          }
          event "Set Gate Widths": Value Change {
            # "Frechem: Did not change"
            n150 = event-data() -> ()  [unwired: 2 out]
            n151 = local read "Current"() -> (w372:dbl[unit])
            n152 = local read "Gate Width: Time / Percent"() -> (w366:bool)
            n153 = call "gate percent to width.vi"("Trigger Freq"=w372, "Gate %"="Target") -> ("Gate width"=w368:dbl[unit])  [unwired: 1 out]
            n154 = call "gate percent to width.vi"("Trigger Freq"=w372, "Gate %"="Target") -> ("Gate width"=w367:dbl[unit])  [unwired: 1 out]
            n155 = Select(t=w368, s=w366, f=w359) -> (s? t:f=w369:dbl[unit])
            n156 = Select(t=w367, s=w366, f=w360) -> (s? t:f=w365:dbl[unit])
            n157 = call "Set both gates.vi"("Error In"=w377, "VISA resource name"=w378, "Set Width?"=TRUE, "Gate B Width"=w365, "Gate A Width"=w369) -> ("Error Out"=w381:errorcluster, "VISA resource name out"=w380:refnum<visa-resource-name>)  [unwired: 3 in, 2 out]
            n158 = call "Read both gates.vi"("error in (no error)"=w381, "VISA resource name"=w380) -> ("Gate B Width"=w361:dbl[unit], "Gate A Width"=w362:dbl[unit], "error out"=w375:errorcluster, "VISA resource name out"=w376:refnum<visa-resource-name>)  [unwired: 6 out]
            n159 = local write "Current"(w362) -> ()
            n160 = local write "Current"(w361) -> ()
            n161 = call "gate width to percent.vi"("Trigger Freq"=w372, "Gate width"=w362) -> ("Gate %"=w373:dbl)  [unwired: 1 out]
            n162 = call "gate width to percent.vi"("Trigger Freq"=w372, "Gate width"=w361) -> ("Gate %"=w374:dbl)  [unwired: 1 out]
            n163 = local write "Actual"(w373) -> ()
            n164 = local write "Actual"(w374) -> ()
            n165 = Bundle By Name(cluster=w364, "Gate A Width"=w362, "Gate B Width"=w361) -> (w363:T3)
          }
          event "Set Gate Mode": Value Change {
            # "Frechem: Did not change"
            n166 = event-data() -> ()  [unwired: 7 out]
            n167 = local write "Current"(w383) -> ()
            n168 = local write "Current"(w382) -> ()
            n169 = Bundle By Name(cluster=w385, "Gate A Mode"=w382, "Gate B Mode"=w383) -> (w384:T3)
            n170 = call "Set gate mode.vi"("error in (no error)"=w390, "Mode (def: CW)"=w382, "Gate (def: A)"=enum16{"Gate A", "Gate B"}."Gate A" ("i (0)"), "VISA resource name"=w391) -> ("error out"=w389:errorcluster, "VISA resource name out"=w388:refnum<visa-resource-name>)  [unwired: 6 out]
            n171 = call "Set gate mode.vi"("error in (no error)"=w389, "Mode (def: CW)"=w383, "Gate (def: A)"=enum16{"Gate A", "Gate B"}."Gate B" ("i (0)"), "VISA resource name"=w388) -> ("error out"=w387:errorcluster, "VISA resource name out"=w386:refnum<visa-resource-name>)  [unwired: 6 out]
          }
          event "Internal / External", "# Triggers vs Freq/Time": Value Change {
            # "Frechem: Did not change"
            n172 = event-data() -> ()  [unwired: 2 out]
            n173 = property on="Update visible/hidden" class="Bool (strict)"("Val(Sgnl)"=TRUE ("Value (Signaling)")) -> ()  [unwired: 2 in, 2 out]
          }
          event "Gate Width: Time / Percent": Value Change {
            # "Frechem: Did not change"
            # "Changes the gate widths to percents and updates values.\n\"Current\" is the value last read from the device."
            n174 = event-data() -> ("NewVal"=w402:bool)  [unwired: 6 out]
            n175 = local read "Current"() -> (w403:dbl[unit])
            n176 = property on="Update visible/hidden" class="Bool (strict)"("Val(Sgnl)"=TRUE ("Value (Signaling)")) -> ()  [unwired: 2 in, 2 out]
            n177 = case shown="True" w402 {
              tunnel: w403 -> [w408 w424]
              tunnel: [w405 w415] -> w399
              tunnel: w398 -> [w405 w415]
              frame False {
                n178 = local read "Actual"() -> (w411:dbl)
                n179 = local read "Actual"() -> (w412:dbl)
                n180 = local read "Target"() -> (w406:dbl)
                n181 = local read "Target"() -> (w407:dbl)
                n182 = call "gate percent to width.vi"("Trigger Freq"=w408, "Gate %"=w411) -> ("Gate width"=w409:dbl[unit])  [unwired: 1 out]
                n183 = call "gate percent to width.vi"("Trigger Freq"=w408, "Gate %"=w412) -> ("Gate width"=w410:dbl[unit])  [unwired: 1 out]
                n184 = call "gate percent to width.vi"("Trigger Freq"=w408, "Gate %"=w406) -> ("Gate width"=w414:dbl[unit])  [unwired: 1 out]
                n185 = call "gate percent to width.vi"("Trigger Freq"=w408, "Gate %"=w407) -> ("Gate width"=w413:dbl[unit])  [unwired: 1 out]
                n186 = local write "Current"(w409) -> ()
                n187 = local write "Current"(w410) -> ()
                n188 = local write "Setpoint"(w414) -> ()
                n189 = local write "Setpoint"(w413) -> ()
              }
              frame True {
                n190 = local read "Setpoint"() -> (w423:dbl[unit])
                n191 = local read "Setpoint"() -> (w421:dbl[unit])
                n192 = local read "Current"() -> (w419:dbl[unit])
                n193 = local read "Current"() -> (w417:dbl[unit])
                n194 = call "gate width to percent.vi"("Trigger Freq"=w424, "Gate width"=w423) -> ("Gate %"=w422:dbl)  [unwired: 1 out]
                n195 = call "gate width to percent.vi"("Trigger Freq"=w424, "Gate width"=w421) -> ("Gate %"=w420:dbl)  [unwired: 1 out]
                n196 = call "gate width to percent.vi"("Trigger Freq"=w424, "Gate width"=w419) -> ("Gate %"=w418:dbl)  [unwired: 1 out]
                n197 = call "gate width to percent.vi"("Trigger Freq"=w424, "Gate width"=w417) -> ("Gate %"=w416:dbl)  [unwired: 1 out]
                n198 = local write "Target"(w422) -> ()
                n199 = local write "Target"(w420) -> ()
                n200 = local write "Actual"(w418) -> ()
                n201 = local write "Actual"(w416) -> ()
              }
            }
          }
          event "Start / Middle": Value Change {
            # "Frechem: Did not change"
            # "Updates the gate widths depending on when it is set."
            n202 = event-data() -> ("NewVal"=w428:bool)  [unwired: 6 out]
            n203 = case shown="False" w428 {
              frame False {
                n204 = local read "Current"() -> (w442:dbl[unit])
                n205 = local read "Current"() -> (w439:dbl[unit])
                n206 = local read "Setpoint"() -> (w437:dbl[unit])
                n207 = local read "Setpoint"() -> (w432:dbl[unit])
                n208 = local read "Current"() -> (w435:dbl[unit])
                n209 = local read "Current"() -> (w430:dbl[unit])
                n210 = Divide(x=w442, y=2) -> (x/y=w438:dbl[unit])
                n211 = Divide(x=w439, y=2) -> (x/y=w433:dbl[unit])
                n212 = Subtract(x=w435, y=w438) -> (x-y=w434:dbl[unit])
                n213 = Subtract(x=w437, y=w438) -> (x-y=w436:dbl[unit])
                n214 = Subtract(x=w430, y=w433) -> (x-y=w429:dbl[unit])
                n215 = Subtract(x=w432, y=w433) -> (x-y=w431:dbl[unit])
                n216 = local write "Current"(w434) -> ()
                n217 = local write "Setpoint"(w436) -> ()
                n218 = local write "Current"(w429) -> ()
                n219 = local write "Setpoint"(w431) -> ()
              }
              frame True {
                n220 = local read "Current"() -> (w453:dbl[unit])
                n221 = local read "Current"() -> (w456:dbl[unit])
                n222 = local read "Setpoint"() -> (w446:dbl[unit])
                n223 = local read "Setpoint"() -> (w451:dbl[unit])
                n224 = local read "Current"() -> (w444:dbl[unit])
                n225 = local read "Current"() -> (w449:dbl[unit])
                n226 = Divide(x=w453, y=2) -> (x/y=w447:dbl[unit])
                n227 = Divide(x=w456, y=2) -> (x/y=w452:dbl[unit])
                n228 = Add(x=w444, y=w447) -> (x+y=w443:dbl[unit])
                n229 = Add(x=w446, y=w447) -> (x+y=w445:dbl[unit])
                n230 = Add(x=w449, y=w452) -> (x+y=w448:dbl[unit])
                n231 = Add(x=w451, y=w452) -> (x+y=w450:dbl[unit])
                n232 = local write "Current"(w443) -> ()
                n233 = local write "Setpoint"(w445) -> ()
                n234 = local write "Current"(w448) -> ()
                n235 = local write "Setpoint"(w450) -> ()
              }
            }
          }
          event "Update visible/hidden": Value Change {
            n236 = event-data() -> ()  [unwired: 7 out]
            n237 = flat-sequence {
              frame #0 {
                n238 = property on="Target" class="DigNum (strict)"("Visible"="Gate Width: Time / Percent") -> ()  [unwired: 2 in, 2 out]
                n239 = property on="Actual" class="DigNum (strict)"("Visible"="Gate Width: Time / Percent") -> ()  [unwired: 2 in, 2 out]
                n240 = property on="Actual" class="DigNum (strict)"("Visible"="Gate Width: Time / Percent") -> ()  [unwired: 2 in, 2 out]
                n241 = property on="Target" class="DigNum (strict)"("Visible"="Gate Width: Time / Percent") -> ()  [unwired: 2 in, 2 out]
                n242 = Not(x="Gate Width: Time / Percent") -> (.not. x?=w462:bool)
                n243 = property on="Setpoint" class="DigNum (strict)"("Visible"=w462) -> ()  [unwired: 2 in, 2 out]
                n244 = property on="Current" class="DigNum (strict)"("Visible"=w462) -> ()  [unwired: 2 in, 2 out]
                n245 = property on="Current" class="DigNum (strict)"("Visible"=w462) -> ()  [unwired: 2 in, 2 out]
                n246 = property on="Setpoint" class="DigNum (strict)"("Visible"=w462) -> ()  [unwired: 2 in, 2 out]
              }
              frame #1 {
                # "Frechem: Did not change"
                n247 = local read "Internal / External"() -> (w465:bool)
                n248 = local read "# Triggers vs Freq/Time"() -> (w464:bool)
                n249 = Not(x=w465) -> (.not. x?=w463:bool)
                n250 = property on="Set Count Time" class="Bool"("Visible"=w463) -> ()  [unwired: 2 in, 2 out]
                n251 = Or(x=w463, y=w464) -> (x .or. y?=w469:bool)
                n252 = Not(x=w464) -> (.not. x?=w466:bool)
                n253 = And(x=w465, y=w464) -> (x .and. y?=w468:bool)
                n254 = property on="Setpoint" class="DigNum (strict)"("Visible"=w468) -> ()  [unwired: 2 in, 2 out]
                n255 = property on="Current" class="DigNum (strict)"("Visible"=w468) -> ()  [unwired: 2 in, 2 out]
                n256 = property on="Current" class="DigNum (strict)"("Visible"=w469) -> ()  [unwired: 2 in, 2 out]
                n257 = property on="Setpoint" class="DigNum (strict)"("Visible"=w469) -> ()  [unwired: 2 in, 2 out]
                n258 = And(x=w465, y=w466) -> (x .and. y?=w467:bool)
                n259 = property on="Set Time & Freq." class="Bool"("Visible"=w468) -> ()  [unwired: 2 in, 2 out]
                n260 = property on="Setpoint" class="DigNum (strict)"("Visible"=w467) -> ()  [unwired: 2 in, 2 out]
                n261 = property on="Current" class="DigNum (strict)"("Visible"=w467) -> ()  [unwired: 2 in, 2 out]
                n262 = property on="# Triggers vs Freq/Time" class="Bool (strict)"("Visible"=w465) -> ()  [unwired: 2 in, 2 out]
                n263 = property on="Set # of Triggers" class="Bool"("Visible"=w467) -> ()  [unwired: 2 in, 2 out]
              }
            }
            n264 = local write "Update visible/hidden"(FALSE ("Update visiible/hidden")) -> ()
          }
          event "Set # Periods": Value Change {
            # "This allows you to update the number of periods to be taken while the device is running\nwithout being reinitialized."
            n265 = event-data() -> ()  [unwired: 2 out]
            n266 = call "Set Num Periods.vi"("# of periods"=w470, "Set # Periods"="Set # Periods", "Error In"=w472, "VISA resource name"=w473) -> ("Error Out"=w479:errorcluster, "VISA resource name out"=w478:refnum<visa-resource-name>)  [unwired: 6 in]
            n267 = call "Get Number Periods.vi"("error in (no error)"=w479, "VISA resource name"=w478) -> ("error out"=w474:errorcluster, "# Periods"=→"Current":dbl, "VISA resource name out"=w475:refnum<visa-resource-name>)  [unwired: 7 in]
          }
          event "Set Dwell Time": Value Change {
            # "This allows you to update the dwell time\nwithout reinitialization."
            n268 = event-data() -> ()  [unwired: 7 out]
            n269 = call "Set Dwell Time.vi"("Error In"=w488, "Dwell time"=w486, "Set # Periods"="Set Dwell Time", "VISA resource name"=w489) -> ("Error Out"=w484:errorcluster, "VISA resource name out"=w485:refnum<visa-resource-name>)  [unwired: 6 in]
            n270 = call "Get Dwell Time.vi"("error in (no error)"=w484, "VISA resource name"=w485) -> ("error out"=w481:errorcluster, "output"=→"Current":dbl[unit], "VISA resource name out"=w482:refnum<visa-resource-name>)  [unwired: 7 in]
          }
          event "Read Buffer Data": Value Change {
            # "Read data VI courtesy of Paul Henning on the\nNational Instruments forum."
            n271 = event-data() -> ()  [unwired: 7 out]
            n272 = Add(x=w493, y=w492) -> (x+y=w490:dbl[unit])
            n273 = flat-sequence {
              tunnel: w504 -> [w516]
              tunnel: w506 -> [w515]
              tunnel: w508 -> [w514]
              tunnel: w510 -> [w513]
              tunnel: [w513] -> w503
              tunnel: [w514] -> w502
              tunnel: [w515] -> w501
              tunnel: [w516] -> w500
              tunnel: [w512] -> w495
              tunnel: w494 -> [w512]
              tunnel: [w511] -> w491
              tunnel: w490 -> [w511]
              tunnel: w503 -> [w526]
              tunnel: w502 -> [w524]
              tunnel: w501 -> [w522]
              tunnel: w500 -> [w520]
              tunnel: [w525] -> w499
              tunnel: [w523] -> w498
              tunnel: [w521] -> w497
              tunnel: w495 -> [w518]
              tunnel: w491 -> [w517]
              tunnel: [w569] -> w505
              tunnel: [w566] -> w507
              tunnel: [w567] -> w509
              tunnel: w499 -> [w564]
              tunnel: w498 -> [w568]
              tunnel: w497 -> [w569]
              frame #0 {
              }
              frame #1 {
                n274 = case shown="True" TRUE {
                  tunnel: w526 -> [w527 w538]
                  tunnel: [w527 w537] -> w525
                  tunnel: w524 -> [w528 w536]
                  tunnel: [w528 w535] -> w523
                  tunnel: w522 -> [w529 w534]
                  tunnel: [w529 w533] -> w521
                  tunnel: w520 -> [_ w532]
                  tunnel: w518 -> [_ w531]
                  tunnel: w517 -> [_ w530]
                  frame False {
                  }
                  frame True {
                    n275 = flat-sequence {
                      tunnel: w532 -> [w557]
                      tunnel: w538 -> [w540]
                      tunnel: w536 -> [w555]
                      tunnel: w534 -> [w556]
                      tunnel: w531 -> [w553]
                      tunnel: [w539] -> w537
                      tunnel: [w555] -> w535
                      tunnel: [w556] -> w533
                      tunnel: w530 -> [w551]
                      frame #0 {
                        n276 = Index Array(array=w553, index=0) -> (element=w550:timestamp)
                        n277 = Number To Decimal String(number="GPIB Address") -> (decimal integer string=w561:string)  [unwired: 1 in]
                        n278 = call "Read Data.vi"("Channel Number"=1, "GPIB Address"=w561, "Number of Datapoints"=w557) -> ("Data"=w554:i32[])
                        n279 = call "Read Data.vi"("Channel Number"=0, "GPIB Address"=w561, "Number of Datapoints"=w557) -> ("Data"=w545:i32[])
                        n280 = node(w551) -> (w542:dbl)
                        n281 = Bundle By Name("Y"=w554, "t0"=w550, "dt"=w542) -> (w543:waveform(i32))  [unwired: 1 in]
                        n282 = To Double Precision Float(number=w545) -> (double precision float=w544:dbl[])
                        n283 = Bundle By Name("Y"=w544, "t0"=w550, "dt"=w542) -> (w549:waveform(dbl))  [unwired: 1 in]
                        n284 = Build Array(w549, w543) -> (w548:waveform(dbl)[])
                        n285 = call-poly <vilib>:"Export Waveforms to Spreadsheet File.vi"("header? (write header:T)"=FALSE, "error in (no error)"=w540, "multiple time columns? (single:F)"=FALSE, "waveforms"=w548, "file path (dialog if empty)"="file path") -> ("error out"=w539:errorcluster)  [unwired: 5 in, 1 out]
                      }
                    }
                  }
                }
              }
              frame #2 {
                w562 = dbl[] [] ("History Data")
                n286 = property on="Counter A" class="WFChart (strict)"(error in=w564, "History Data"=w562) -> (error out=w563:errorcluster)  [unwired: 1 in, 1 out]
                n287 = property on="Counter B" class="WFChart (strict)"(error in=w563, "History Data"=w562) -> (error out=w565:errorcluster)  [unwired: 1 in, 1 out]
                n288 = call "Reset Counters.vi"("error in (no error)"=w565, "VISA resource name"=w568) -> ("error out"=w567:errorcluster, "VISA resource name out"=w566:refnum<visa-resource-name>)  [unwired: 8 in]
              }
            }
            n289 = local write "Read Buffer Data"(FALSE ("Read Buffer Data")) -> ()
          }
          event "Start Scan": Value Change {
            # "This allows you to start and stop a scan with the counts being from the buffer for display."
            n290 = event-data() -> ()  [unwired: 7 out]
            n291 = flat-sequence {
              tunnel: w591 -> [w863]
              tunnel: w590 -> [w858]
              tunnel: w589 -> [w859]
              tunnel: [w861] -> w600
              tunnel: [w862] -> w599
              tunnel: [w863] -> w598
              tunnel: [w868] -> w597
              tunnel: [w866] -> w596
              tunnel: [w865] -> w595
              tunnel: w600 -> [w869]
              tunnel: w599 -> [w867]
              tunnel: w598 -> [w865]
              tunnel: [w871] -> w593
              tunnel: w597 -> [w871]
              tunnel: w596 -> [w870]
              tunnel: [w872] -> w592
              tunnel: w595 -> [w872]
              tunnel: [w870] -> w594
              frame #0 {
                n292 = call "Clear Status Byte.vi"("error in (no error)"=w859, "VISA resource name"=w858) -> ("error out"=w860:errorcluster, "VISA resource name out"=w857:refnum<visa-resource-name>)  [unwired: 8 in]
                n293 = call "Reset Counters.vi"("error in (no error)"=w860, "VISA resource name"=w857) -> ("error out"=w861:errorcluster, "VISA resource name out"=w862:refnum<visa-resource-name>)  [unwired: 8 in]
              }
              frame #1 {
                n294 = call "Start button.vi"("error in (no error)"=w869, "VISA resource name"=w867) -> ("error out"=w868:errorcluster, "VISA resource name out"=w866:refnum<visa-resource-name>)  [unwired: 8 in]
                n295 = Get Date/Time In Seconds() -> (seconds since 1Jan1904=→"Scan Start Time":timestamp)
              }
              frame #2 {
                n296 = local write "Start Scan"(FALSE ("Read Channels")) -> ()
              }
            }
            n297 = call <vilib>:"DAQmx Start Task.vi"("task/channels in"=w575) -> ("task out"=w574:refnum<k21>)  [unwired: 13 in, 1 out]
            n298 = call <vilib>:"DAQmx Start Task.vi"("task/channels in"=w573) -> ("task out"=w572:refnum<k21>)  [unwired: 13 in, 1 out]
            n299 = while {
              tunnel: [w640] -> w587
              tunnel: w594 -> [w635]
              tunnel: [w641] -> w586
              tunnel: w593 -> [w636]
              tunnel: [w642] -> w588
              tunnel: w592 -> [w639]
              tunnel: [w637] -> w585
              shift-right: [w633] -> _
              shift-left: 0.0 -> [w601]
              tunnel: w582 -> [w632]
              tunnel: w583 -> [w625]
              shift-right: [w623] -> w580
              shift-left: w581 -> [w622]
              tunnel: w574 -> [w620]
              tunnel: [w618] -> w570
              tunnel: w579 -> [w617]
              shift-right: [w606] -> _
              shift-left: dbl[] [] ("data") -> [w614]
              shift-right: [w613] -> _
              shift-left: 0.0 -> [w615]
              shift-right: [w608] -> _
              shift-left: 0.0 -> [w609]
              tunnel: w572 -> [w605]
              tunnel: [w602] -> w571
              stop <- w628 stop-if-true
              n300 = flat-sequence {
                tunnel: w635 -> [w659]
                tunnel: [w659] -> w646
                tunnel: w636 -> [w658]
                tunnel: [w658] -> w645
                tunnel: w639 -> [w657]
                tunnel: [w657] -> w638
                tunnel: ["Stop Scan"] -> w629
                tunnel: [w655] -> w626
                tunnel: w625 -> [w655]
                tunnel: [w654] -> w621
                tunnel: w620 -> [w654]
                tunnel: w615 -> [w653]
                tunnel: w614 -> [w650]
                tunnel: [w652] -> w611
                tunnel: [w651] -> w610
                tunnel: w609 -> [w651]
                tunnel: w605 -> [w647]
                tunnel: [w647] -> w604
                tunnel: [w682] -> w644
                tunnel: w646 -> [w684]
                tunnel: w645 -> [w683]
                tunnel: [w688] -> w643
                tunnel: w638 -> [w688]
                tunnel: [w681] -> w634
                tunnel: w601 -> [w680]
                tunnel: [w679] -> w627
                tunnel: w626 -> [w677]
                tunnel: [w676] -> w624
                tunnel: w622 -> [w675]
                tunnel: w621 -> [w673]
                tunnel: [w672] -> w619
                tunnel: w617 -> [w671]
                tunnel: [w670] -> w616
                tunnel: [w669] -> w612
                tunnel: w611 -> [w667]
                tunnel: w610 -> [w665]
                tunnel: [w664] -> w607
                tunnel: w604 -> [w662]
                tunnel: [w661] -> w603
                tunnel: w601 -> [w660]
                tunnel: [w833] -> w642
                tunnel: [w832] -> w641
                tunnel: w644 -> [w837]
                tunnel: w643 -> [w836]
                tunnel: [w835] -> w640
                tunnel: w628 -> [w838]
                tunnel: [w831] -> w637
                tunnel: w634 -> [w834]
                tunnel: [w830] -> w633
                tunnel: w627 -> [w830]
                tunnel: w624 -> [w829]
                tunnel: [w829] -> w623
                tunnel: w619 -> [w826]
                tunnel: [w826] -> w618
                tunnel: w616 -> [w823]
                tunnel: [w825] -> w613
                tunnel: w612 -> [w825]
                tunnel: [w824] -> w608
                tunnel: w607 -> [w824]
                tunnel: [w822] -> w606
                tunnel: w603 -> [w820]
                tunnel: [w820] -> w602
                frame #0 {
                  n301 = Index Array(array=w650, index=0) -> (element=w648:dbl)
                  n302 = Add(x=w648, y=w653) -> (x+y=w652:dbl)
                }
                frame #1 {
                  n303 = flat-sequence {
                    tunnel: w683 -> [w696]
                    tunnel: w684 -> [w695]
                    tunnel: [w699] -> w687
                    tunnel: [w697] -> w686
                    tunnel: [w694] -> w685
                    tunnel: [w693] -> w678
                    tunnel: w677 -> [w693]
                    tunnel: [w692] -> w674
                    tunnel: w673 -> [w692]
                    tunnel: [w691] -> w668
                    tunnel: w667 -> [w691]
                    tunnel: [w690] -> w666
                    tunnel: w665 -> [w690]
                    tunnel: [w689] -> w663
                    tunnel: w662 -> [w689]
                    tunnel: w687 -> [w719]
                    tunnel: w686 -> [w718]
                    tunnel: w685 -> [w720]
                    tunnel: w680 -> [w715]
                    tunnel: [w717] -> w681
                    tunnel: [w716] -> w682
                    tunnel: [w714] -> w679
                    tunnel: w678 -> [w713]
                    tunnel: [w712] -> w676
                    tunnel: w675 -> [w711]
                    tunnel: w674 -> [w710]
                    tunnel: [w709] -> w672
                    tunnel: w671 -> [w708]
                    tunnel: [w707] -> w670
                    tunnel: [w706] -> w669
                    tunnel: w668 -> [w705]
                    tunnel: w666 -> [w704]
                    tunnel: [w703] -> w664
                    tunnel: w663 -> [w702]
                    tunnel: [w701] -> w661
                    tunnel: w660 -> [w700]
                    frame #0 {
                      n304 = call "Query Status Byte.vi"("error in (no error)"=w696, "VISA resource name"=w695) -> ("error out"=w697:errorcluster, "Status Register"=w698:T6, "VISA resource name out"=w699:refnum<visa-resource-name>)  [unwired: 7 in]
                      n305 = Unbundle(w698) -> ("Data Ready"=w694:bool)  [unwired: 10 out]
                    }
                    frame #1 {
                      n306 = case shown="True" w720 {
                        tunnel: w719 -> [w733 w761]
                        tunnel: w718 -> [w732 w760]
                        tunnel: [w732 w758] -> w716
                        tunnel: [w733 w759] -> w717
                        tunnel: w715 -> [w731 w757]
                        tunnel: [w731 w756] -> w714
                        tunnel: w713 -> [_ w755]
                        tunnel: [w730 w754] -> w712
                        tunnel: w711 -> [w730 w753]
                        tunnel: w710 -> [w723 w752]
                        tunnel: [w722 w751] -> w709
                        tunnel: w708 -> [w729 _]
                        tunnel: [w728 _] -> w707
                        tunnel: [w727 _] -> w706
                        tunnel: w705 -> [w727 w750]
                        tunnel: w704 -> [w726 w749]
                        tunnel: [w724 _] -> w703
                        tunnel: w702 -> [w721 w748]
                        tunnel: [w721 w747] -> w701
                        tunnel: w700 -> [_ w734]
                        frame False {
                          n307 = Add(x=1.0, y=w726) -> (x+y=w724:dbl)
                          n308 = call-poly <vilib>:"DAQmx Read.vi"("task/channels in"=w723, "number of samples per channel"=w729) -> ("task out"=w722:refnum<k21>, "data"=w728:dbl[][])  [unwired: 11 in, 1 out]
                        }
                        frame True {
                          n309 = flat-sequence {
                            tunnel: w761 -> [w782]
                            tunnel: w760 -> [w781]
                            tunnel: [w778] -> w746
                            tunnel: [w776] -> w745
                            tunnel: [w772] -> w744
                            tunnel: w755 -> [w772]
                            tunnel: [w771] -> w743
                            tunnel: w752 -> [w770]
                            tunnel: [w769] -> w742
                            tunnel: w750 -> [w766]
                            tunnel: w749 -> [w767]
                            tunnel: w748 -> [w762]
                            tunnel: [w762] -> w741
                            tunnel: w746 -> [w794]
                            tunnel: [w794] -> w740
                            tunnel: w745 -> [w793]
                            tunnel: [w793] -> w739
                            tunnel: w744 -> [w792]
                            tunnel: [w792] -> w738
                            tunnel: w743 -> [w791]
                            tunnel: [w791] -> w737
                            tunnel: w742 -> [w790]
                            tunnel: [w790] -> w736
                            tunnel: w741 -> [w788]
                            tunnel: [w789] -> w735
                            tunnel: w734 -> [w787]
                            tunnel: [w818] -> w758
                            tunnel: [w819] -> w759
                            tunnel: w740 -> [w816]
                            tunnel: w739 -> [w817]
                            tunnel: w757 -> [w814]
                            tunnel: [w813] -> w756
                            tunnel: w738 -> [_]
                            tunnel: w737 -> [w812]
                            tunnel: [w811] -> w754
                            tunnel: w753 -> [w810]
                            tunnel: w736 -> [w809]
                            tunnel: [w809] -> w751
                            tunnel: [w808] -> w747
                            tunnel: w735 -> [w808]
                            frame #0 {
                              n310 = call "Query Counts.vi"("error in (no error)"=w781, "Read B?"=FALSE, "VISA resource name"=w782) -> ("error out"=w777:errorcluster, "Counts"=→"Counter A":dbl, "VISA resource name out"=w779:refnum<visa-resource-name>)  [unwired: 6 in]
                              n311 = call-poly <vilib>:"DAQmx Read.vi"("task/channels in"=w770) -> ("task out"=w769:refnum<k21>, "data"=w765:dbl[])  [unwired: 12 in, 1 out]
                              n312 = call "Query Counts.vi"("error in (no error)"=w777, "Read B?"=TRUE, "VISA resource name"=w779) -> ("error out"=w776:errorcluster, "Counts"=→"Counter B":dbl, "VISA resource name out"=w778:refnum<visa-resource-name>)  [unwired: 6 in]
                              n313 = Index Array(array=w765, index=0) -> (element=→"Wavemeter":dbl)
                              n314 = Divide(x=w766, y=w767) -> (x/y=→"PMT":dbl)
                              n315 = Get Date/Time In Seconds() -> (seconds since 1Jan1904=w771:timestamp)
                            }
                            frame #1 {
                              n316 = Quotient & Remainder(x=w787, y=2.0) -> (x-y*floor(x/y)=w784:dbl)  [unwired: 1 out]
                              n317 = Equal?(x=w784, y=0.0) -> (x = y?=w783:bool)
                              "Trigger" <- w783
                              n318 = case shown="False" w783 {
                                tunnel: [w795 w799] -> w789
                                tunnel: w788 -> [w795 w798]
                                frame False {
                                }
                                frame True {
                                n319 = flat-sequence {
                                tunnel: w798 -> [w801]
                                tunnel: [w800] -> w796
                                tunnel: [w803] -> w797
                                tunnel: w796 -> [w803]
                                tunnel: [w806] -> w799
                                tunnel: w797 -> [w805]
                                frame #0 {
                                n320 = call-poly <vilib>:"DAQmx Write.vi"("task/channels in"=w801, "data"=5.0) -> ("task out"=w800:refnum<k21>)  [unwired: 11 in, 2 out]
                                }
                                frame #1 {
                                n321 = Wait (ms)(milliseconds to wait=u32 1) -> ()  [unwired: 1 out]
                                }
                                frame #2 {
                                n322 = call-poly <vilib>:"DAQmx Write.vi"("task/channels in"=w805, "data"=0.0) -> ("task out"=w806:refnum<k21>)  [unwired: 11 in, 2 out]
                                }
                                }
                                }
                              }
                            }
                            frame #2 {
                              n323 = Build Array (concatenate)(w810, w812) -> (w811:timestamp[])
                              n324 = call "Clear Status Byte.vi"("error in (no error)"=w817, "VISA resource name"=w816) -> ("error out"=w818:errorcluster, "VISA resource name out"=w819:refnum<visa-resource-name>)  [unwired: 8 in]
                              n325 = Add(x=w814, y=1.0) -> (x+y=w813:dbl)
                            }
                          }
                        }
                      }
                    }
                  }
                }
                frame #2 {
                  n326 = case shown="True" w838 {
                    tunnel: w837 -> [w845 w854]
                    tunnel: w834 -> [w844 w855]
                    tunnel: w836 -> [w846 w856]
                    tunnel: [w846 w856] -> w835
                    tunnel: [w842 w849] -> w833
                    tunnel: [w843 w850] -> w832
                    tunnel: [w841 w851] -> w831
                    tunnel: [FALSE TRUE] -> w828
                    tunnel: [TRUE FALSE] -> w827
                    frame False {
                      n327 = call "Query Status Byte.vi"("error in (no error)"=w845, "VISA resource name"=w844) -> ("error out"=w842:errorcluster, "Status Register"=w841:T6, "VISA resource name out"=w843:refnum<visa-resource-name>)  [unwired: 7 in]
                    }
                    frame True {
                      n328 = call "Stop button.vi"("error in (no error)"=w854, "VISA resource name"=w855) -> ("error out"=w852:errorcluster, "VISA resource name out"=w853:refnum<visa-resource-name>)  [unwired: 8 in]
                      n329 = call "Query Status Byte.vi"("error in (no error)"=w852, "VISA resource name"=w853) -> ("error out"=w849:errorcluster, "Status Register"=w851:T6, "VISA resource name out"=w850:refnum<visa-resource-name>)  [unwired: 7 in]
                    }
                  }
                  "Scan Finished" <- w828
                  "Scanning" <- w827
                  n330 = Index Array(array=w823, index (row)=1) -> (element=w822:dbl[])  [unwired: 1 in]
                }
              }
              n331 = To Double Precision Float(number=w632) -> (double precision float=w631:dbl)
              n332 = Equal?(x=w601, y=w631) -> (x = y?=w630:bool)
              n333 = Or(x=w629, y=w630) -> (x .or. y?=w628:bool)
              "Current Period" <- w601
            }
          }
        }
        n334 = call <vilib>:"Simple Error Handler.vi"("error in (no error)"=w59) -> ("error out"=w58:errorcluster)  [unwired: 1 in, 7 out]
      }
      n335 = call <vilib>:"DAQmx Wait Until Done.vi"("task/channels in"=w23, "timeout (sec)"=w24) -> ("task out"=w25:refnum<k21>)  [unwired: 12 in, 1 out]
      n336 = call <vilib>:"DAQmx Wait Until Done.vi"("task/channels in"=w21, "timeout (sec)"=w24) -> ("task out"=w22:refnum<k21>)  [unwired: 12 in, 1 out]
      n337 = call <vilib>:"DAQmx Clear Task.vi"("task in"=w25) -> ()  [unwired: 14 in, 1 out]
      n338 = call <vilib>:"DAQmx Clear Task.vi"("task in"=w22) -> ()  [unwired: 14 in, 1 out]
    }
    frame #2 {
    }
  }
  "error out" <- w6
